vi "test_Update CD XML File.vi"(8 "error in (no error)":errorcluster, 11 "TestCase in":refnum<class "LVLIBP CD XML Updater Unit Tests.lvclass">) -> (0 "error out":errorcluster, 3 "TestCase out":refnum<class "LVLIBP CD XML Updater Unit Tests.lvclass">)   [LabVIEW 2018, in "LVLIBP CD XML Updater Unit Tests.lvclass"]
uses:
  LVLIBP CD XML Updater Unit Tests.lvclass
  <vilib>/addons/_JKI Toolkits/VI Tester/TestCase.llb/TestCase.lvclass
  Utilities/.LVLIBP CD XML Updater/.LVLIBP CD XML Updater.lvlib
  Utilities/.LVLIBP CD XML Updater/Project XML Editor/Project XML Editor.lvclass
  FPGA Addon Test Class/FPGA Addon Test Class.lvclass
  C:/Program Files (x86)/National Instruments/LabVIEW 2018/vi.lib/addons/_JKI Toolkits/VI Tester/TestCase.llb/TestCase.lvclass
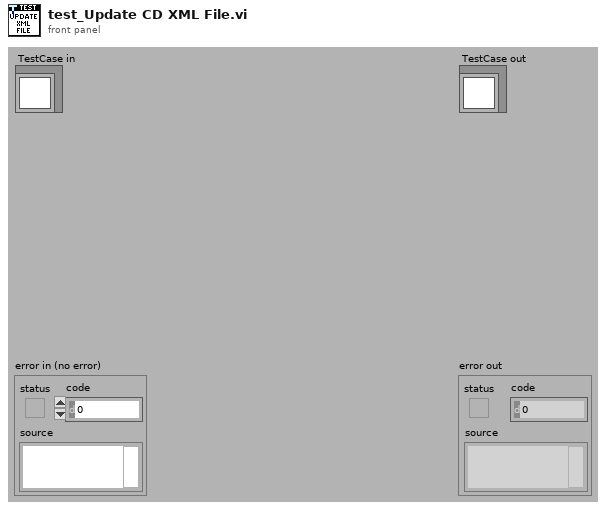
[diagram p1: front panel]
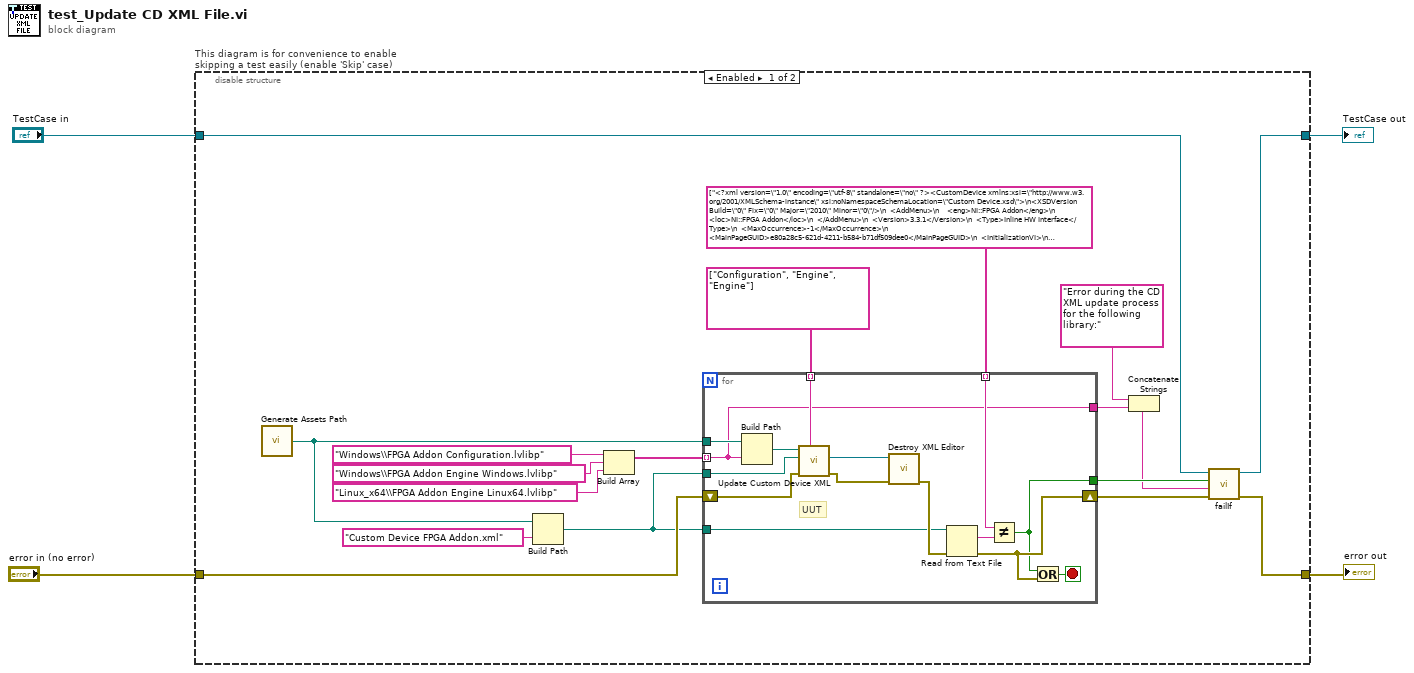
[diagram p0: block diagram]
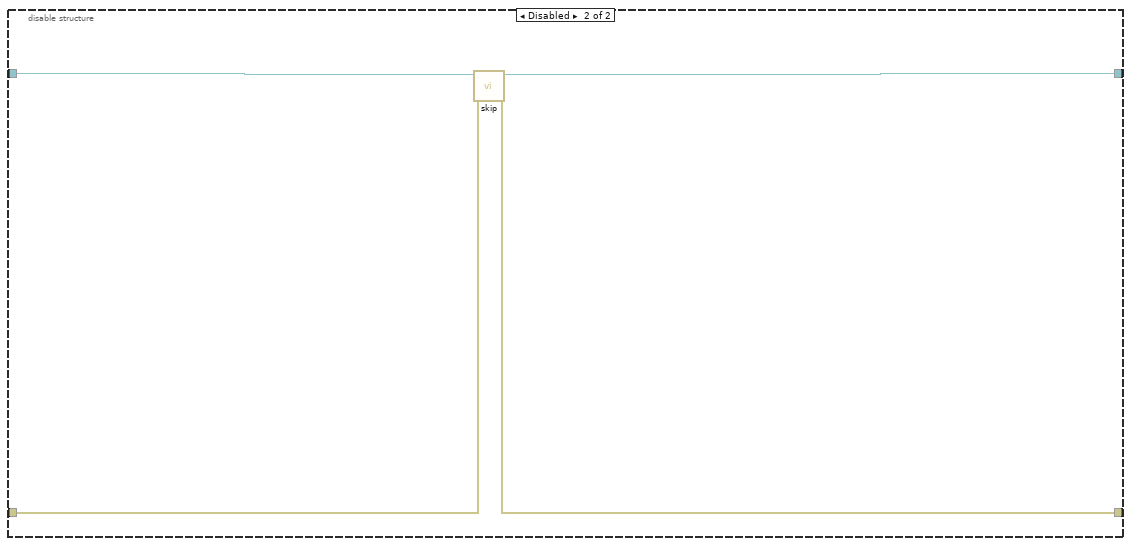
[diagram p2: hidden frame]
diagram:
  n1 = disable-structure "This diagram is for convenience to enable skipping a test easily (enable 'Skip' case)" shown="Enabled" {
    disable-tunnel: "TestCase in" -> [w16 w41]
    disable-tunnel: [w15 w39] -> w1
    disable-tunnel: [w6 w40] -> w3
    disable-tunnel: "error in (no error)" -> [w9 w38]
    frame Enabled {
      n2 = call "Generate Assets Path.vi"() -> ("Assets path"=w11:path)
      n3 = Build Path(base path=w11, name or relative path="Custom Device FPGA Addon.xml") -> (appended path=w5:path)
      n4 = Build Array("Windows\\FPGA Addon Configuration.lvlibp" ("name or relative path"), "Windows\\FPGA Addon Engine Windows.lvlibp" ("name or relative path"), "Linux_x64\\FPGA Addon Engine Linux64.lvlibp" ("name or relative path")) -> (w10:string[])
      n5 = for {
        tunnel: string[] ["Configuration", "Engine", "Engine"] -> [w37] mode=indexing
        tunnel: w5 -> [w36]
        shift-right: [w30] -> w7
        shift-left: w9 -> [w29]
        tunnel: string[] ["<?xml version=\"1.0\" encoding=\"utf-8\" standalone=\"no\" ?><CustomDevice xmlns:xsi=\"http://www.w3.org/2001/XMLSchema-instance\" xsi:noNamespaceSchemaLocation=\"Custom Device.xsd\">\n<XSDVersion Build=\"0\" Fix=\"0\" Major=\"2010\" Minor=\"0\"/>\n  <AddMenu>\n    <eng>NI::FPGA Addon</eng>\n    <loc>NI::FPGA Addon</loc>\n  </AddMenu>\n  <Version>3.3.1</Version>\n  <Type>Inline HW Interface</Type>\n  <MaxOccurrence>-1</MaxOccurrence>\n  <MainPageGUID>e80a28c5-621d-4211-b584-b71df509dee0</MainPageGUID>\n  <InitializationVI>\n    <Type>Action</Type>\n    <Item2Launch>\n      <Type>To Common Doc Dir</Type>\n\t\t<Path>Custom Devices\\FPGA Addon\\Windows\\FPGA Addon Configuration.lvlibp\\Addon\\Addon System Explorer\\Initialization VI.vi</Path>\n    </Item2Launch>\n  </InitializationVI>\n  <CustomDeviceVI>\n\t<SourceDistribution>\n\t\t<Source>\n\t\t\t<SupportedTarget>Windows</SupportedTarget>\n\t\t\t<Source>\n\t\t\t\t<Type>To Common Doc Dir</Type>\n\t\t\t\t<Path>Custom Devices\\FPGA Addon\\Windows\\FPGA Addon Engine Windows.llb\\RT Driver VI.vi</Path>\n\t\t\t</Source>\n\t\t\t<RealTimeSystemDestination>c:\\ni-rt\\VeriStand\\Custom Devices\\FPGA Addon\\FPGA Addon Engine Windows.llb\\RT Driver VI.vi</RealTimeSystemDestination>\n\t\t</Source>\n\t\t<Source>\n\t\t\t<SupportedTarget>Linux_x64</SupportedTarget>\n\t\t\t<Source>\n\t\t\t\t<Type>To Common Doc Dir</Type>\n\t\t\t\t<Path>Custom Devices\\FPGA Addon\\Linux_x64\\FPGA Addon Engine Linux64.llb\\RT Driver VI.vi</Path>\n\t\t\t</Source>\n\t\t\t<RealTimeSystemDestination>c:\\ni-rt\\VeriStand\\Custom Devices\\FPGA Addon\\FPGA Addon Engine Linux64.llb\\RT Driver VI.vi</RealTimeSystemDestination>\n\t\t</Source>\n\t</SourceDistribution>\n\t</CustomDeviceVI>\n  <Dependencies/>\n  <Pages>\n    <Page>\n      <Name>\n        <eng>FPGA Addon</eng>\n        <loc>FPGA Addon</loc>\n      </Name>\n      <GUID>e80a28c5-621d-4211-b584-b71df509dee0</GUID>\n      <Glyph>\n\t\t  \t<Type>To Application Data Dir</Type>\n\t\t\t  <Path>System Explorer\\Glyphs\\fpga device.png</Path>\n\t\t  </Glyph>\n      <Item2Launch>\n        <Type>To Common Doc Dir</Type>\n\t\t    <Path>Custom Devices\\FPGA Addon\\Windows\\FPGA Addon Configuration.lvlibp\\Addon\\Addon System Explorer\\Main Page.vi</Path>\n      </Item2Launch>\n      <RunTimeMenu>\n        <MenuItem>\n          <GUID>01e8f077-156a-4698-bbdc-a047cf741b9d</GUID>\n          <Type>Action</Type>\n          <Name>\n            <eng>Disable</eng>\n            <loc>Disable</loc>\n          </Name>\n          <Item2Launch>\n            <Type>To Common Doc Dir</Type>\n            <Path>Custom Devices\\FPGA Addon\\Windows\\FPGA Addon Configuration.lvlibp\\Addon\\Addon System Explorer\\RTMs\\EnableDisable Main Page.vi</Path>\n          </Item2Launch>\n        </MenuItem>\n        <MenuItem>\n\t\t\t\t\t<GUID>b2ce9074-10ee-4035-b1de-8d57db17ae03</GUID>\n\t\t\t\t\t<Type>Action</Type>\n\t\t\t\t\t<Name>\n\t\t\t\t\t\t<eng>Export Config</eng>\n\t\t\t\t\t\t<loc>Export Config</loc>\n\t\t\t\t\t</Name>\n\t\t\t\t\t<Item2Launch>\n\t\t\t\t\t\t<Type>To Common Doc Dir</Type>\n\t\t\t\t\t\t<Path>Custom Devices\\FPGA Addon\\Windows\\FPGA Addon Configuration.lvlibp\\Addon\\Addon System Explorer\\RTMs\\ExportConfigurationToFile.vi</Path>\n\t\t\t\t\t</Item2Launch>\n\t\t\t\t</MenuItem>\n        <MenuItem>\n          <GUID>7755077A-1485-13A6-5674A23FB86277FF</GUID>\n          <Type>Separator</Type>\n          <Name>\n            <eng>.</eng>\n            <loc>.</loc>\n          </Name>\n          <Item2Launch>\n            <Type>Absolute</Type>\n            <Path>.</Path>\n          </Item2Launch>\n        </MenuItem>\n        <MenuItem>\n          <GUID>77550670-1485-13A6-568B9AB41979630D</GUID>\n          <Type>Action</Type>\n          <Name>\n            <eng>Delete</eng>\n            <loc>Delete</loc>\n          </Name>\n          <Item2Launch>\n            <Type>Absolute</Type>\n            <Path>Actions\\Delete.vi</Path>\n          </Item2Launch>\n        </MenuItem>\n      </RunTimeMenu>\n      <ActionVIOnLoad>\n        <Type>To Common Doc Dir</Type>\n        <Path>Custom Devices\\FPGA Addon\\Windows\\FPGA Addon Configuration.lvlibp\\Addon\\Addon System Explorer\\Actions\\ActionVIOnLoad.vi</Path>\n      </ActionVIOnLoad>\n      <ActionVIOnCompile>\n        <Type>To Common Doc Dir</Type>\n        <Path>Custom Devices\\FPGA Addon\\Windows\\FPGA Addon Configuration.lvlibp\\Addon\\Addon System Explorer\\Actions\\ActionVIOnCompile.vi</Path>\n      </ActionVIOnCompile>\n    </Page>\n    <Page>\n      <Name>\n        <eng>FPGA Addon</eng>\n        <loc>FPGA Addon</loc>\n      </Name>\n      <GUID>1903f8c0-e426-4f25-b8ca-65973b1160fd</GUID>\n      <Glyph>\n        <Type>To Application Data Dir</Type>\n        <Path>System Explorer\\Glyphs\\fpga device_disabled.png</Path>\n      </Glyph>\n      <Item2Launch>\n        <Type>To Common Doc Dir</Type>\n        <Path>Custom Devices\\FPGA Addon\\Windows\\FPGA Addon Configuration.lvlibp\\Addon\\Addon System Explorer\\Main Page.vi</Path>\n      </Item2Launch>\n      <RunTimeMenu>\n        <MenuItem>\n          <GUID>01e8f077-156a-4698-bbdc-a047cf741b9d</GUID>\n          <Type>Action</Type>\n          <Name>\n            <eng>Enable</eng>\n            <loc>Enable</loc>\n          </Name>\n          <Item2Launch>\n            <Type>To Common Doc Dir</Type>\n            <Path>Custom Devices\\FPGA Addon\\Windows\\FPGA Addon Configuration.lvlibp\\Addon\\Addon System Explorer\\RTMs\\EnableDisable Main Page.vi</Path>\n          </Item2Launch>\n        </MenuItem>\n        <MenuItem>\n          <GUID>b2ce9074-10ee-4035-b1de-8d57db17ae03</GUID>\n          <Type>Action</Type>\n          <Name>\n            <eng>Export Config</eng>\n            <loc>Export Config</loc>\n          </Name>\n          <Item2Launch>\n            <Type>To Common Doc Dir</Type>\n            <Path>Custom Devices\\FPGA Addon\\Windows\\FPGA Addon Configuration.lvlibp\\Addon\\Addon System Explorer\\RTMs\\ExportConfigurationToFile.vi</Path>\n          </Item2Launch>\n        </MenuItem>\n        <MenuItem>\n          <GUID>7755077A-1485-13A6-5674A23FB86277FF</GUID>\n          <Type>Separator</Type>\n          <Name>\n            <eng>.</eng>\n            <loc>.</loc>\n          </Name>\n          <Item2Launch>\n            <Type>Absolute</Type>\n            <Path>.</Path>\n          </Item2Launch>\n        </MenuItem>\n        <MenuItem>\n          <GUID>77550670-1485-13A6-568B9AB41979630D</GUID>\n          <Type>Action</Type>\n          <Name>\n            <eng>Delete</eng>\n            <loc>Delete</loc>\n          </Name>\n          <Item2Launch>\n            <Type>Absolute</Type>\n            <Path>Actions\\Delete.vi</Path>\n          </Item2Launch>\n        </MenuItem>\n      </RunTimeMenu>\n      <ActionVIOnLoad>\n        <Type>To Common Doc Dir</Type>\n        <Path>Custom Devices\\FPGA Addon\\Windows\\FPGA Addon Configuration.lvlibp\\Addon\\Addon System Explorer\\Actions\\ActionVIOnLoad.vi</Path>\n      </ActionVIOnLoad>\n    </Page>\n    <Page>\n      <Name>\n        <eng>Scalars</eng>\n        <loc>Scalars</loc>\n      </Name>\n      <DisallowRenaming>true</DisallowRenaming>\n      <DeleteProtection>true</DeleteProtection>\n      <GUID>884b7050-623e-4f2c-925b-6b753ddf9d1a</GUID>\n      <Glyph>\n\t\t  \t<Type>To Application Data Dir</Type>\n\t\t\t  <Path>System Explorer\\Glyphs\\default fpga channel.png</Path>\n\t\t  </Glyph>\n      <Item2Launch>\n        <Type>To Common Doc Dir</Type>\n\t\t    <Path>Custom Devices\\FPGA Addon\\Windows\\FPGA Addon Configuration.lvlibp\\Addon\\Addon System Explorer\\Extra Pages\\Scalars.vi</Path>\n      </Item2Launch>\n      <RunTimeMenu>\n        <MenuItem>\n          <GUID>03D3BE0A-1485-13A6-563AEB9BF271825A</GUID>\n          <Type>VI</Type>\n          <MinNrOfChilds>1</MinNrOfChilds>\n          <Name>\n            <eng>Delete Multiple Items</eng>\n            <loc>Delete Multiple Items</loc>\n          </Name>\n          <Item2Launch>\n            <Type>Absolute</Type>\n            <Path>Dialogs\\Delete Multiple Items.vi</Path>\n          </Item2Launch>\n        </MenuItem>    \n      </RunTimeMenu>\n    </Page>\n    <Page>\n      <Name>\n        <eng>Scalar Inputs</eng>\n        <loc>Scalar Inputs</loc>\n      </Name>\n      <DisallowRenaming>true</DisallowRenaming>\n      <DeleteProtection>true</DeleteProtection>\n      <GUID>45f50bc5-dab3-4e15-b99b-0f8c8c0fe0f0</GUID>\n      <Glyph>\n\t\t  \t<Type>To Application Data Dir</Type>\n\t\t  \t<Path>System Explorer\\Glyphs\\ChnGroup.png</Path>\n\t\t  </Glyph>\n      <Item2Launch>\n        <Type>To Common Doc Dir</Type>\n\t\t    <Path>Custom Devices\\FPGA Addon\\Windows\\FPGA Addon Configuration.lvlibp\\Addon\\Addon System Explorer\\Extra Pages\\Scalar Inputs.vi</Path>\n      </Item2Launch>\n    </Page>\n    <Page>\n      <Name>\n        <eng>Group Input</eng>\n        <loc>Group Input</loc>\n      </Name>\n      <GUID>88748f7d-ce11-4328-8f35-56fd574a40c1</GUID>\n      <Glyph>\n        <Type>To Common Doc Dir</Type>\n\t\t    <Path>Custom Devices\\FPGA Addon\\Windows\\Glyphs\\Group.png</Path>\n\t\t  </Glyph>\n      <Item2Launch>\n        <Type>To Common Doc Dir</Type>\n\t\t    <Path>Custom Devices\\FPGA Addon\\Windows\\FPGA Addon Configuration.lvlibp\\Addon\\Addon System Explorer\\Extra Pages\\Scalar Inputs.vi</Path>\n      </Item2Launch>\n    </Page>\n    <Page>\n      <Name>\n        <eng>Scalar Outputs</eng>\n        <loc>Scalar Outputs</loc>\n      </Name>\n      <DisallowRenaming>true</DisallowRenaming>\n      <DeleteProtection>true</DeleteProtection>\n      <GUID>7d46fed9-731a-4423-8f13-aa8ac2cd791c</GUID>\n      <Glyph>\n\t\t\t  <Type>To Application Data Dir</Type>\n\t\t\t  <Path>System Explorer\\Glyphs\\ChnGroup.png</Path>\n\t\t  </Glyph>\n      <Item2Launch>\n        <Type>To Common Doc Dir</Type>\n\t\t    <Path>Custom Devices\\FPGA Addon\\Windows\\FPGA Addon Configuration.lvlibp\\Addon\\Addon System Explorer\\Extra Pages\\Scalar Outputs.vi</Path>\n      </Item2Launch>\n    </Page>\n    <Page>\n      <Name>\n        <eng>Group Output</eng>\n        <loc>Group Output</loc>\n      </Name>\n      <GUID>58901a15-a42e-477a-af06-3ceeb84f52de</GUID>\n      <Glyph>\n        <Type>To Common Doc Dir</Type>\n\t\t    <Path>Custom Devices\\FPGA Addon\\Windows\\Glyphs\\Group.png</Path>\n\t\t  </Glyph>\n      <Item2Launch>\n        <Type>To Common Doc Dir</Type>\n\t\t    <Path>Custom Devices\\FPGA Addon\\Windows\\FPGA Addon Configuration.lvlibp\\Addon\\Addon System Explorer\\Extra Pages\\Scalar Outputs.vi</Path>\n      </Item2Launch>\n    </Page>\n    <Page>\n      <Name>\n        <eng>Waveforms</eng>\n        <loc>Waveforms</loc>\n      </Name>\n      <DisallowRenaming>true</DisallowRenaming>\n      <DeleteProtection>true</DeleteProtection>\n      <GUID>5f75895a-bfdb-4cd8-9ef2-787e261eba38</GUID>\n      <Glyph>\n\t\t\t  <Type>To Application Data Dir</Type>\n\t\t\t  <Path>System Explorer\\Glyphs\\waveform.png</Path>\n\t\t  </Glyph>\n      <Item2Launch>\n        <Type>To Common Doc Dir</Type>\n\t\t    <Path>Custom Devices\\FPGA Addon\\Windows\\FPGA Addon Configuration.lvlibp\\Addon\\Addon System Explorer\\Extra Pages\\Waveforms.vi</Path>\n      </Item2Launch>\n      <RunTimeMenu>\n        <MenuItem>\n          <GUID>03D3BE0A-1485-13A6-563AEB9BF271825A</GUID>\n          <Type>VI</Type>\n          <MinNrOfChilds>1</MinNrOfChilds>\n          <Name>\n            <eng>Delete Multiple Items</eng>\n            <loc>Delete Multiple Items</loc>\n          </Name>\n          <Item2Launch>\n            <Type>Absolute</Type>\n            <Path>Dialogs\\Delete Multiple Items.vi</Path>\n          </Item2Launch>\n        </MenuItem>\n      </RunTimeMenu>\n    </Page>\n    <Page>\n      <Name>\n        <eng>Waveform Inputs</eng>\n        <loc>Waveform Inputs</loc>\n      </Name>\n      <DisallowRenaming>true</DisallowRenaming>\n      <DeleteProtection>true</DeleteProtection>\n      <ExcludeFromAlphabeticalOrder>true</ExcludeFromAlphabeticalOrder>\n      <GUID>165959cb-b691-43bd-9f8b-54fe62f4b534</GUID>\n      <Glyph>\n\t\t\t  <Type>To Application Data Dir</Type>\n\t\t\t  <Path>System Explorer\\Glyphs\\ChnGroup.png</Path>\n\t\t  </Glyph>\n      <Item2Launch>\n        <Type>To Common Doc Dir</Type>\n\t\t    <Path>Custom Devices\\FPGA Addon\\Windows\\FPGA Addon Configuration.lvlibp\\Addon\\Addon System Explorer\\Extra Pages\\Waveform Inputs.vi</Path>\n      </Item2Launch>\n    </Page>\n    <Page>\n      <Name>\n        <eng>Waveform Outputs</eng>\n        <loc>Waveform Outputs</loc>\n      </Name>\n      <DisallowRenaming>true</DisallowRenaming>\n      <DeleteProtection>true</DeleteProtection>\n      <ExcludeFromAlphabeticalOrder>true</ExcludeFromAlphabeticalOrder>\n      <GUID>bc66db3e-ace6-4d58-add4-89e89e885df7</GUID>\n      <Glyph>\n        <Type>To Application Data Dir</Type>\n        <Path>System Explorer\\Glyphs\\ChnGroup.png</Path>\n      </Glyph>\n      <Item2Launch>\n        <Type>To Common Doc Dir</Type>\n        <Path>Custom Devices\\FPGA Addon\\Windows\\FPGA Addon Configuration.lvlibp\\Addon\\Addon System Explorer\\Extra Pages\\Waveform Outputs.vi</Path>\n      </Item2Launch>\n    </Page>\n    <Page>\n      <Name>\n        <eng>Scalar Input</eng>\n        <loc>Scalar Input</loc>\n      </Name>\n      <GUID>9bd0c044-925c-4d1d-a44e-de3c4043858c</GUID>\n      <Glyph>\n\t\t  \t<Type>To Application Data Dir</Type>\n\t\t  \t<Path>System Explorer\\Glyphs\\default fpga channel.png</Path>\n\t\t  </Glyph>\n      <Item2Launch>\n        <Type>To Common Doc Dir</Type>\n\t\t    <Path>Custom Devices\\FPGA Addon\\Windows\\FPGA Addon Configuration.lvlibp\\Addon\\Addon System Explorer\\Extra Pages\\Scalar Input.vi</Path>\n      </Item2Launch>\n      <RunTimeMenu>\n        <MenuItem>\n          <GUID>2cd33a82-ccc0-4cb3-affc-1385b5dc0dd8</GUID>\n          <Type>Action</Type>\n          <Name>\n            <eng>Enable Bitpacked</eng>\n            <loc>Enable Bitpacked</loc>\n          </Name>\n          <Item2Launch>\n            <Type>To Common Doc Dir</Type>\n            <Path>Custom Devices\\FPGA Addon\\Windows\\FPGA Addon Configuration.lvlibp\\Addon\\Addon System Explorer\\RTMs\\Switch Scalar Type.vi</Path>\n          </Item2Launch>\n        </MenuItem>\n        <MenuItem>\n          <GUID>7755077A-1485-13A6-5674A23FB86277FF</GUID>\n          <Type>Separator</Type>\n          <Name>\n            <eng>.</eng>\n            <loc>.</loc>\n          </Name>\n          <Item2Launch>\n            <Type>Absolute</Type>\n            <Path>.</Path>\n          </Item2Launch>\n        </MenuItem>\n        <MenuItem>\n          <GUID>77550670-1485-13A6-568B9AB41979630D</GUID>\n          <Type>Action</Type>\n          <Name>\n            <eng>Delete</eng>\n            <loc>Delete</loc>\n          </Name>\n          <Item2Launch>\n            <Type>Absolute</Type>\n            <Path>Actions\\Delete.vi</Path>\n          </Item2Launch>\n        </MenuItem>\n      </RunTimeMenu>\n    </Page>\n    <Page>\n      <Name>\n        <eng>Scalar Output</eng>\n        <loc>Scalar Output</loc>\n      </Name>\n      <GUID>625afbbf-e929-46eb-93d1-fe7033ba1e7b</GUID>\n      <Glyph>\n\t\t  \t<Type>To Application Data Dir</Type>\n\t\t  \t<Path>System Explorer\\Glyphs\\default fpga channel.png</Path>\n\t  \t</Glyph>\n      <Item2Launch>\n        <Type>To Common Doc Dir</Type>\n\t\t    <Path>Custom Devices\\FPGA Addon\\Windows\\FPGA Addon Configuration.lvlibp\\Addon\\Addon System Explorer\\Extra Pages\\Scalar Output.vi</Path>\n      </Item2Launch>\n      <RunTimeMenu>\n        <MenuItem>\n          <GUID>2cd33a82-ccc0-4cb3-affc-1385b5dc0dd8</GUID>\n          <Type>Action</Type>\n          <Name>\n            <eng>Enable Bitpacked</eng>\n            <loc>Enable Bitpacked</loc>\n          </Name>\n          <Item2Launch>\n            <Type>To Common Doc Dir</Type>\n            <Path>Custom Devices\\FPGA Addon\\Windows\\FPGA Addon Configuration.lvlibp\\Addon\\Addon System Explorer\\RTMs\\Switch Scalar Type.vi</Path>\n          </Item2Launch>\n        </MenuItem>\n        <MenuItem>\n          <GUID>7755077A-1485-13A6-5674A23FB86277FF</GUID>\n          <Type>Separator</Type>\n          <Name>\n            <eng>.</eng>\n            <loc>.</loc>\n          </Name>\n          <Item2Launch>\n            <Type>Absolute</Type>\n            <Path>.</Path>\n          </Item2Launch>\n        </MenuItem>\n        <MenuItem>\n          <GUID>77550670-1485-13A6-568B9AB41979630D</GUID>\n          <Type>Action</Type>\n          <Name>\n            <eng>Delete</eng>\n            <loc>Delete</loc>\n          </Name>\n          <Item2Launch>\n            <Type>Absolute</Type>\n            <Path>Actions\\Delete.vi</Path>\n          </Item2Launch>\n        </MenuItem>\n      </RunTimeMenu>\n    </Page>\n    <Page>\n      <Name>\n        <eng>DMA</eng>\n        <loc>DMA</loc>\n      </Name>\n      <ExcludeFromAlphabeticalOrder>true</ExcludeFromAlphabeticalOrder>\n      <GUID>fdfaa619-d09f-452b-8143-c1a261c13b7a</GUID>\n      <Glyph>\n\t\t\t  <Type>To Application Data Dir</Type>\n\t\t\t  <Path>System Explorer\\Glyphs\\Lookup Table.png</Path>\n\t\t  </Glyph>\n      <Item2Launch>\n        <Type>To Common Doc Dir</Type>\n\t\t    <Path>Custom Devices\\FPGA Addon\\Windows\\FPGA Addon Configuration.lvlibp\\Addon\\Addon System Explorer\\Extra Pages\\DMA Channel.vi</Path>\n      </Item2Launch>\n      <RunTimeMenu>\n         <MenuItem>\n            <GUID>345ad323-e622-4d27-9f97-b3d588c29827</GUID>\n            <Type>Action</Type>\n            <Name>\n              <eng>Import DMA Channels</eng>\n              <loc>Import DMA Channels</loc>\n            </Name>\n            <Item2Launch>\n              <Type>To Common Doc Dir</Type>\n              <Path>Custom Devices\\FPGA Addon\\Windows\\FPGA Addon Configuration.lvlibp\\Addon\\Addon System Explorer\\RTMs\\Import DMA Channels RTM.vi</Path>\n            </Item2Launch>\n          </MenuItem>\n          <MenuItem>\n            <GUID>7755077A-1485-13A6-5674A23FB86277FF</GUID>\n            <Type>Separator</Type>\n            <Name>\n              <eng>.</eng>\n              <loc>.</loc>\n            </Name>\n            <Item2Launch>\n              <Type>Absolute</Type>\n              <Path>.</Path>\n            </Item2Launch>\n          </MenuItem>\n      </RunTimeMenu>\n    <ButtonList>\n        <Button>\n          <ID>Import DMA Channels</ID>\n          <Glyph>\n            <Type>To Application Data Dir</Type>\n            <Path>System Explorer\\Glyphs\\NI-XNET ImportXNETFrames.png</Path>\n          </Glyph>\n          <Type>Action</Type>\n          <ReferencedGUID>345ad323-e622-4d27-9f97-b3d588c29827</ReferencedGUID>\n          <ButtonText>\n            <eng>Import DMA Channels</eng>\n            <loc>Import DMA Channels</loc>\n          </ButtonText>\n          <Caption>\n            <eng>Import DMA Channels</eng>\n            <loc>Import DMA Channels</loc>\n          </Caption>\n          <TipStrip>\n            <eng>Import DMA Channels</eng>\n            <loc>Import DMA Channels</loc>\n          </TipStrip>\n          <Documentation>\n            <eng/>\n            <loc/>\n          </Documentation>\n        </Button>\n    </ButtonList>\n    </Page>\n    <Page>\n      <Name>\n        <eng>Waveform Output</eng>\n        <loc>Waveform Output</loc>\n      </Name>\n      <DeleteProtection>true</DeleteProtection>\n      <ExcludeFromAlphabeticalOrder>true</ExcludeFromAlphabeticalOrder>\n      <GUID>0c0ecc88-7768-47db-a589-856e32a93156</GUID>\n      <Glyph>\n        <Type>To Application Data Dir</Type>\n        <Path>System Explorer\\Glyphs\\waveform.png</Path>\n      </Glyph>\n      <Item2Launch>\n        <Type>To Common Doc Dir</Type>\n        <Path>Custom Devices\\FPGA Addon\\Windows\\FPGA Addon Configuration.lvlibp\\Addon\\Addon System Explorer\\Extra Pages\\Waveform Output.vi</Path>\n      </Item2Launch>\n    </Page>\n    <Page>\n      <Name>\n        <eng>Waveform Input</eng>\n        <loc>Waveform Input</loc>\n      </Name>\n      <DeleteProtection>true</DeleteProtection>\n      <ExcludeFromAlphabeticalOrder>true</ExcludeFromAlphabeticalOrder>\n      <GUID>2afc1de4-b056-47bb-a2ad-eec5ad0d30b6</GUID>\n      <Glyph>\n        <Type>To Application Data Dir</Type>\n        <Path>System Explorer\\Glyphs\\waveform.png</Path>\n      </Glyph>\n      <Item2Launch>\n        <Type>To Common Doc Dir</Type>\n        <Path>Custom Devices\\FPGA Addon\\Windows\\FPGA Addon Configuration.lvlibp\\Addon\\Addon System Explorer\\Extra Pages\\Waveform Input.vi</Path>\n      </Item2Launch>\n    </Page>\n    <Page>\n      <Name>\n        <eng>DMA Status Channels</eng>\n        <loc>DMA Status Channels</loc>\n      </Name>\n      <DisallowRenaming>true</DisallowRenaming>\n      <DeleteProtection>true</DeleteProtection>\n      <ExcludeFromAlphabeticalOrder>true</ExcludeFromAlphabeticalOrder>\n      <GUID>4e1a084b-2b8b-4128-8417-f0007d9ffe93</GUID>\n      <Glyph>\n\t\t  \t<Type>To Application Data Dir</Type>\n\t\t  \t<Path>System Explorer\\Glyphs\\event-based.png</Path>\n\t\t  </Glyph>\n      <Item2Launch>\n        <Type>To Common Doc Dir</Type>\n\t    \t<Path>Custom Devices\\FPGA Addon\\Windows\\FPGA Addon Configuration.lvlibp\\Addon\\Addon System Explorer\\Extra Pages\\DMA Status Channels.vi</Path>\n      </Item2Launch>\n    </Page>\n    <Page>\n      <Name>\n        <eng>DMA Error</eng>\n        <loc>DMA Error</loc>\n      </Name>\n      <DisallowRenaming>true</DisallowRenaming>\n      <DeleteProtection>true</DeleteProtection>\n      <GUID>708ff167-b4eb-405e-bb0f-5c2fb305da21</GUID>\n      <Glyph>\n        <Type>To Application Data Dir</Type>\n        <Path>System Explorer\\Glyphs\\RM Information Channels.png</Path>\n      </Glyph>\n      <Item2Launch>\n        <Type>To Common Doc Dir</Type>\n        <Path>Custom Devices\\FPGA Addon\\Windows\\FPGA Addon Configuration.lvlibp\\Addon\\Addon System Explorer\\Extra Pages\\DMA Error.vi</Path>\n      </Item2Launch>\n    </Page>\n    <Page>\n      <Name>\n        <eng>DMA Elements Remaining</eng>\n        <loc>DMA Elements Remaining</loc>\n      </Name>\n      <DisallowRenaming>true</DisallowRenaming>\n      <DeleteProtection>true</DeleteProtection>\n      <GUID>785497d1-fc1e-46c9-8feb-aa61f2850cff</GUID>\n      <Glyph>\n        <Type>To Application Data Dir</Type>\n        <Path>System Explorer\\Glyphs\\RM Information Channels.png</Path>\n      </Glyph>\n      <Item2Launch>\n        <Type>To Common Doc Dir</Type>\n        <Path>Custom Devices\\FPGA Addon\\Windows\\FPGA Addon Configuration.lvlibp\\Addon\\Addon System Explorer\\Extra Pages\\DMA Elements Remaining.vi</Path>\n      </Item2Launch>\n    </Page>\n    <Page>\n      <Name>\n        <eng>Scalar Input Bitpacked</eng>\n        <loc>Scalar Input Bitpacked</loc>\n      </Name>\n      <ExcludeFromAlphabeticalOrder>true</ExcludeFromAlphabeticalOrder>\n      <GUID>8489bf21-57e3-4e68-bdd5-eadff573ec1e</GUID>\n      <Glyph>\n        <Type>To Common Doc Dir</Type>\n\t\t  <Path>Custom Devices\\FPGA Addon\\Windows\\Glyphs\\Bitpacked.png</Path>\n      </Glyph>\n      <Item2Launch>\n        <Type>To Common Doc Dir</Type>\n        <Path>Custom Devices\\FPGA Addon\\Windows\\FPGA Addon Configuration.lvlibp\\Addon\\Addon System Explorer\\Extra Pages\\Scalar Bitpacked.vi</Path>\n      </Item2Launch>\n      <RunTimeMenu>\n        <MenuItem>\n          <GUID>2cd33a82-ccc0-4cb3-affc-1385b5dc0dd8</GUID>\n          <Type>Action</Type>\n          <Name>\n            <eng>Disable Bitpacked</eng>\n            <loc>Disable Bitpacked</loc>\n          </Name>\n          <Item2Launch>\n            <Type>To Common Doc Dir</Type>\n            <Path>Custom Devices\\FPGA Addon\\Windows\\FPGA Addon Configuration.lvlibp\\Addon\\Addon System Explorer\\RTMs\\Switch Scalar Type.vi</Path>\n          </Item2Launch>\n        </MenuItem>\n        <MenuItem>\n          <GUID>7755077A-1485-13A6-5674A23FB86277FF</GUID>\n          <Type>Separator</Type>\n          <Name>\n            <eng>.</eng>\n            <loc>.</loc>\n          </Name>\n          <Item2Launch>\n            <Type>Absolute</Type>\n            <Path>.</Path>\n          </Item2Launch>\n        </MenuItem>\n        <MenuItem>\n          <GUID>77550670-1485-13A6-568B9AB41979630D</GUID>\n          <Type>Action</Type>\n          <Name>\n            <eng>Delete</eng>\n            <loc>Delete</loc>\n          </Name>\n          <Item2Launch>\n            <Type>Absolute</Type>\n            <Path>Actions\\Delete.vi</Path>\n          </Item2Launch>\n        </MenuItem>\n      </RunTimeMenu>\n    </Page>\n    <Page>\n      <Name>\n        <eng>Scalar Output Bitpacked</eng>\n        <loc>Scalar Output Bitpacked</loc>\n      </Name>\n      <ExcludeFromAlphabeticalOrder>true</ExcludeFromAlphabeticalOrder>\n      <GUID>ebfc3e29-7579-49df-b828-0da2c3787b5f</GUID>\n      <Glyph>\n        <Type>To Common Doc Dir</Type>\n\t\t  <Path>Custom Devices\\FPGA Addon\\Windows\\Glyphs\\Bitpacked.png</Path>\n      </Glyph>\n      <Item2Launch>\n        <Type>To Common Doc Dir</Type>\n        <Path>Custom Devices\\FPGA Addon\\Windows\\FPGA Addon Configuration.lvlibp\\Addon\\Addon System Explorer\\Extra Pages\\Scalar Bitpacked.vi</Path>\n      </Item2Launch>\n      <RunTimeMenu>\n        <MenuItem>\n          <GUID>2cd33a82-ccc0-4cb3-affc-1385b5dc0dd8</GUID>\n          <Type>Action</Type>\n          <Name>\n            <eng>Disable Bitpacked</eng>\n            <loc>Disable Bitpacked</loc>\n          </Name>\n          <Item2Launch>\n            <Type>To Common Doc Dir</Type>\n            <Path>Custom Devices\\FPGA Addon\\Windows\\FPGA Addon Configuration.lvlibp\\Addon\\Addon System Explorer\\RTMs\\Switch Scalar Type.vi</Path>\n          </Item2Launch>\n        </MenuItem>\n        <MenuItem>\n          <GUID>7755077A-1485-13A6-5674A23FB86277FF</GUID>\n          <Type>Separator</Type>\n          <Name>\n            <eng>.</eng>\n            <loc>.</loc>\n          </Name>\n          <Item2Launch>\n            <Type>Absolute</Type>\n            <Path>.</Path>\n          </Item2Launch>\n        </MenuItem>\n        <MenuItem>\n          <GUID>77550670-1485-13A6-568B9AB41979630D</GUID>\n          <Type>Action</Type>\n          <Name>\n            <eng>Delete</eng>\n            <loc>Delete</loc>\n          </Name>\n          <Item2Launch>\n            <Type>Absolute</Type>\n            <Path>Actions\\Delete.vi</Path>\n          </Item2Launch>\n        </MenuItem>\n      </RunTimeMenu>\n    </Page>\n    <Page>\n      <Name>\n        <eng>Bitpacked Input</eng>\n        <loc>Bitpacked Input</loc>\n      </Name>\n      <DeleteProtection>true</DeleteProtection>\n      <ExcludeFromAlphabeticalOrder>true</ExcludeFromAlphabeticalOrder>\n      <GUID>4b03cffd-e469-431a-ba96-aca85ece66af</GUID>\n      <Glyph>\n        <Type>To Application Data Dir</Type>\n        <Path>System Explorer\\Glyphs\\default fpga channel.png</Path>\n      </Glyph>\n      <Item2Launch>\n        <Type>To Common Doc Dir</Type>\n        <Path>Custom Devices\\FPGA Addon\\Windows\\FPGA Addon Configuration.lvlibp\\Addon\\Addon System Explorer\\Extra Pages\\Scalar Input.vi</Path>\n      </Item2Launch>\n    </Page>\n    <Page>\n      <Name>\n        <eng>Bitpacked Output</eng>\n        <loc>Bitpacked Output</loc>\n      </Name>\n      <DeleteProtection>true</DeleteProtection>\n      <ExcludeFromAlphabeticalOrder>true</ExcludeFromAlphabeticalOrder>\n      <GUID>6db3f02b-654f-4ed6-bd84-80bb5242a557</GUID>\n      <Glyph>\n        <Type>To Application Data Dir</Type>\n        <Path>System Explorer\\Glyphs\\default fpga channel.png</Path>\n      </Glyph>\n      <Item2Launch>\n        <Type>To Common Doc Dir</Type>\n        <Path>Custom Devices\\FPGA Addon\\Windows\\FPGA Addon Configuration.lvlibp\\Addon\\Addon System Explorer\\Extra Pages\\Scalar Output.vi</Path>\n      </Item2Launch>\n    </Page>\n      <Page>\n      <Name>\n        <eng>Static Scalar Input</eng>\n        <loc>Static Scalar Input</loc>\n      </Name>\n      <GUID>7579cb69-d559-4b2b-a1fc-0d112e8661b6</GUID>\n      <Glyph>\n        <Type>To Application Data Dir</Type>\n        <Path>System Explorer\\Glyphs\\default fpga channel.png</Path>\n      </Glyph>\n      <Item2Launch>\n        <Type>To Common Doc Dir</Type>\n        <Path>Custom Devices\\FPGA Addon\\Windows\\FPGA Addon Configuration.lvlibp\\Addon\\Addon System Explorer\\Extra Pages\\Scalar Input.vi</Path>\n      </Item2Launch>\n      <RunTimeMenu>\n        <MenuItem>\n          <GUID>77550670-1485-13A6-568B9AB41979630D</GUID>\n          <Type>Action</Type>\n          <Name>\n            <eng>Delete</eng>\n            <loc>Delete</loc>\n          </Name>\n          <Item2Launch>\n            <Type>Absolute</Type>\n            <Path>Actions\\Delete.vi</Path>\n          </Item2Launch>\n        </MenuItem>\n      </RunTimeMenu>\n    </Page>\n    <Page>\n      <Name>\n        <eng>Static Scalar Output</eng>\n        <loc>Static Scalar Output</loc>\n      </Name>\n      <GUID>ddc5186b-4b14-4629-b48a-cef4575f789c</GUID>\n      <Glyph>\n        <Type>To Application Data Dir</Type>\n        <Path>System Explorer\\Glyphs\\default fpga channel.png</Path>\n      </Glyph>\n      <Item2Launch>\n        <Type>To Common Doc Dir</Type>\n        <Path>Custom Devices\\FPGA Addon\\Windows\\FPGA Addon Configuration.lvlibp\\Addon\\Addon System Explorer\\Extra Pages\\Scalar Output.vi</Path>\n      </Item2Launch>\n      <RunTimeMenu>\n        <MenuItem>\n          <GUID>77550670-1485-13A6-568B9AB41979630D</GUID>\n          <Type>Action</Type>\n          <Name>\n            <eng>Delete</eng>\n            <loc>Delete</loc>\n          </Name>\n          <Item2Launch>\n            <Type>Absolute</Type>\n            <Path>Actions\\Delete.vi</Path>\n          </Item2Launch>\n        </MenuItem>\n      </RunTimeMenu>\n    </Page>\n      <Page>\n      <Name>\n        <eng>Speciality IO</eng>\n        <loc>Speciality IO</loc>\n      </Name>\n      <ExcludeFromAlphabeticalOrder>true</ExcludeFromAlphabeticalOrder>\n      <GUID>25832021-24b6-475a-aa84-f4ed7870ed99</GUID>\n      <Glyph>\n        <Type>To Common Doc Dir</Type>\n\t\t  <Path>Custom Devices\\FPGA Addon\\Windows\\Glyphs\\IP Core.png</Path>\n      </Glyph>\n      <Item2Launch>\n        <Type>To Common Doc Dir</Type>\n        <Path>Custom Devices\\FPGA Addon\\Windows\\FPGA Addon Configuration.lvlibp\\Addon\\Addon System Explorer\\Extra Pages\\Speciality IO.vi</Path>\n      </Item2Launch>\n    </Page>\n  </Pages>\n  <CustomXML>\n    <Dummy/>\n  </CustomXML>\n</CustomDevice>", "<?xml version=\"1.0\" encoding=\"utf-8\" standalone=\"no\" ?><CustomDevice xmlns:xsi=\"http://www.w3.org/2001/XMLSchema-instance\" xsi:noNamespaceSchemaLocation=\"Custom Device.xsd\">\n<XSDVersion Build=\"0\" Fix=\"0\" Major=\"2010\" Minor=\"0\"/>\n  <AddMenu>\n    <eng>NI::FPGA Addon</eng>\n    <loc>NI::FPGA Addon</loc>\n  </AddMenu>\n  <Version>3.3.1</Version>\n  <Type>Inline HW Interface</Type>\n  <MaxOccurrence>-1</MaxOccurrence>\n  <MainPageGUID>e80a28c5-621d-4211-b584-b71df509dee0</MainPageGUID>\n  <InitializationVI>\n    <Type>Action</Type>\n    <Item2Launch>\n      <Type>To Common Doc Dir</Type>\n\t\t<Path>Custom Devices\\FPGA Addon\\Windows\\FPGA Addon Configuration.lvlibp\\Addon\\Addon System Explorer\\Initialization VI.vi</Path>\n    </Item2Launch>\n  </InitializationVI>\n  <CustomDeviceVI>\n\t<SourceDistribution>\n\t\t<Source>\n\t\t\t<SupportedTarget>Windows</SupportedTarget>\n\t\t\t<Source>\n\t\t\t\t<Type>To Common Doc Dir</Type>\n\t\t\t\t<Path>Custom Devices\\FPGA Addon\\Windows\\FPGA Addon Engine Windows.lvlibp\\Addon\\Addon Engine\\RT Driver VI.vi</Path>\n\t\t\t</Source>\n\t\t\t<RealTimeSystemDestination>c:\\ni-rt\\VeriStand\\Custom Devices\\FPGA Addon\\FPGA Addon Engine Windows.lvlibp\\Addon\\Addon Engine\\RT Driver VI.vi</RealTimeSystemDestination>\n\t\t</Source>\n\t\t<Source>\n\t\t\t<SupportedTarget>Linux_x64</SupportedTarget>\n\t\t\t<Source>\n\t\t\t\t<Type>To Common Doc Dir</Type>\n\t\t\t\t<Path>Custom Devices\\FPGA Addon\\Linux_x64\\FPGA Addon Engine Linux64.llb\\RT Driver VI.vi</Path>\n\t\t\t</Source>\n\t\t\t<RealTimeSystemDestination>c:\\ni-rt\\VeriStand\\Custom Devices\\FPGA Addon\\FPGA Addon Engine Linux64.llb\\RT Driver VI.vi</RealTimeSystemDestination>\n\t\t</Source>\n\t</SourceDistribution>\n\t</CustomDeviceVI>\n  <Dependencies/>\n  <Pages>\n    <Page>\n      <Name>\n        <eng>FPGA Addon</eng>\n        <loc>FPGA Addon</loc>\n      </Name>\n      <GUID>e80a28c5-621d-4211-b584-b71df509dee0</GUID>\n      <Glyph>\n\t\t  \t<Type>To Application Data Dir</Type>\n\t\t\t  <Path>System Explorer\\Glyphs\\fpga device.png</Path>\n\t\t  </Glyph>\n      <Item2Launch>\n        <Type>To Common Doc Dir</Type>\n\t\t    <Path>Custom Devices\\FPGA Addon\\Windows\\FPGA Addon Configuration.lvlibp\\Addon\\Addon System Explorer\\Main Page.vi</Path>\n      </Item2Launch>\n      <RunTimeMenu>\n        <MenuItem>\n          <GUID>01e8f077-156a-4698-bbdc-a047cf741b9d</GUID>\n          <Type>Action</Type>\n          <Name>\n            <eng>Disable</eng>\n            <loc>Disable</loc>\n          </Name>\n          <Item2Launch>\n            <Type>To Common Doc Dir</Type>\n            <Path>Custom Devices\\FPGA Addon\\Windows\\FPGA Addon Configuration.lvlibp\\Addon\\Addon System Explorer\\RTMs\\EnableDisable Main Page.vi</Path>\n          </Item2Launch>\n        </MenuItem>\n        <MenuItem>\n\t\t\t\t\t<GUID>b2ce9074-10ee-4035-b1de-8d57db17ae03</GUID>\n\t\t\t\t\t<Type>Action</Type>\n\t\t\t\t\t<Name>\n\t\t\t\t\t\t<eng>Export Config</eng>\n\t\t\t\t\t\t<loc>Export Config</loc>\n\t\t\t\t\t</Name>\n\t\t\t\t\t<Item2Launch>\n\t\t\t\t\t\t<Type>To Common Doc Dir</Type>\n\t\t\t\t\t\t<Path>Custom Devices\\FPGA Addon\\Windows\\FPGA Addon Configuration.lvlibp\\Addon\\Addon System Explorer\\RTMs\\ExportConfigurationToFile.vi</Path>\n\t\t\t\t\t</Item2Launch>\n\t\t\t\t</MenuItem>\n        <MenuItem>\n          <GUID>7755077A-1485-13A6-5674A23FB86277FF</GUID>\n          <Type>Separator</Type>\n          <Name>\n            <eng>.</eng>\n            <loc>.</loc>\n          </Name>\n          <Item2Launch>\n            <Type>Absolute</Type>\n            <Path>.</Path>\n          </Item2Launch>\n        </MenuItem>\n        <MenuItem>\n          <GUID>77550670-1485-13A6-568B9AB41979630D</GUID>\n          <Type>Action</Type>\n          <Name>\n            <eng>Delete</eng>\n            <loc>Delete</loc>\n          </Name>\n          <Item2Launch>\n            <Type>Absolute</Type>\n            <Path>Actions\\Delete.vi</Path>\n          </Item2Launch>\n        </MenuItem>\n      </RunTimeMenu>\n      <ActionVIOnLoad>\n        <Type>To Common Doc Dir</Type>\n        <Path>Custom Devices\\FPGA Addon\\Windows\\FPGA Addon Configuration.lvlibp\\Addon\\Addon System Explorer\\Actions\\ActionVIOnLoad.vi</Path>\n      </ActionVIOnLoad>\n      <ActionVIOnCompile>\n        <Type>To Common Doc Dir</Type>\n        <Path>Custom Devices\\FPGA Addon\\Windows\\FPGA Addon Configuration.lvlibp\\Addon\\Addon System Explorer\\Actions\\ActionVIOnCompile.vi</Path>\n      </ActionVIOnCompile>\n    </Page>\n    <Page>\n      <Name>\n        <eng>FPGA Addon</eng>\n        <loc>FPGA Addon</loc>\n      </Name>\n      <GUID>1903f8c0-e426-4f25-b8ca-65973b1160fd</GUID>\n      <Glyph>\n        <Type>To Application Data Dir</Type>\n        <Path>System Explorer\\Glyphs\\fpga device_disabled.png</Path>\n      </Glyph>\n      <Item2Launch>\n        <Type>To Common Doc Dir</Type>\n        <Path>Custom Devices\\FPGA Addon\\Windows\\FPGA Addon Configuration.lvlibp\\Addon\\Addon System Explorer\\Main Page.vi</Path>\n      </Item2Launch>\n      <RunTimeMenu>\n        <MenuItem>\n          <GUID>01e8f077-156a-4698-bbdc-a047cf741b9d</GUID>\n          <Type>Action</Type>\n          <Name>\n            <eng>Enable</eng>\n            <loc>Enable</loc>\n          </Name>\n          <Item2Launch>\n            <Type>To Common Doc Dir</Type>\n            <Path>Custom Devices\\FPGA Addon\\Windows\\FPGA Addon Configuration.lvlibp\\Addon\\Addon System Explorer\\RTMs\\EnableDisable Main Page.vi</Path>\n          </Item2Launch>\n        </MenuItem>\n        <MenuItem>\n          <GUID>b2ce9074-10ee-4035-b1de-8d57db17ae03</GUID>\n          <Type>Action</Type>\n          <Name>\n            <eng>Export Config</eng>\n            <loc>Export Config</loc>\n          </Name>\n          <Item2Launch>\n            <Type>To Common Doc Dir</Type>\n            <Path>Custom Devices\\FPGA Addon\\Windows\\FPGA Addon Configuration.lvlibp\\Addon\\Addon System Explorer\\RTMs\\ExportConfigurationToFile.vi</Path>\n          </Item2Launch>\n        </MenuItem>\n        <MenuItem>\n          <GUID>7755077A-1485-13A6-5674A23FB86277FF</GUID>\n          <Type>Separator</Type>\n          <Name>\n            <eng>.</eng>\n            <loc>.</loc>\n          </Name>\n          <Item2Launch>\n            <Type>Absolute</Type>\n            <Path>.</Path>\n          </Item2Launch>\n        </MenuItem>\n        <MenuItem>\n          <GUID>77550670-1485-13A6-568B9AB41979630D</GUID>\n          <Type>Action</Type>\n          <Name>\n            <eng>Delete</eng>\n            <loc>Delete</loc>\n          </Name>\n          <Item2Launch>\n            <Type>Absolute</Type>\n            <Path>Actions\\Delete.vi</Path>\n          </Item2Launch>\n        </MenuItem>\n      </RunTimeMenu>\n      <ActionVIOnLoad>\n        <Type>To Common Doc Dir</Type>\n        <Path>Custom Devices\\FPGA Addon\\Windows\\FPGA Addon Configuration.lvlibp\\Addon\\Addon System Explorer\\Actions\\ActionVIOnLoad.vi</Path>\n      </ActionVIOnLoad>\n    </Page>\n    <Page>\n      <Name>\n        <eng>Scalars</eng>\n        <loc>Scalars</loc>\n      </Name>\n      <DisallowRenaming>true</DisallowRenaming>\n      <DeleteProtection>true</DeleteProtection>\n      <GUID>884b7050-623e-4f2c-925b-6b753ddf9d1a</GUID>\n      <Glyph>\n\t\t  \t<Type>To Application Data Dir</Type>\n\t\t\t  <Path>System Explorer\\Glyphs\\default fpga channel.png</Path>\n\t\t  </Glyph>\n      <Item2Launch>\n        <Type>To Common Doc Dir</Type>\n\t\t    <Path>Custom Devices\\FPGA Addon\\Windows\\FPGA Addon Configuration.lvlibp\\Addon\\Addon System Explorer\\Extra Pages\\Scalars.vi</Path>\n      </Item2Launch>\n      <RunTimeMenu>\n        <MenuItem>\n          <GUID>03D3BE0A-1485-13A6-563AEB9BF271825A</GUID>\n          <Type>VI</Type>\n          <MinNrOfChilds>1</MinNrOfChilds>\n          <Name>\n            <eng>Delete Multiple Items</eng>\n            <loc>Delete Multiple Items</loc>\n          </Name>\n          <Item2Launch>\n            <Type>Absolute</Type>\n            <Path>Dialogs\\Delete Multiple Items.vi</Path>\n          </Item2Launch>\n        </MenuItem>    \n      </RunTimeMenu>\n    </Page>\n    <Page>\n      <Name>\n        <eng>Scalar Inputs</eng>\n        <loc>Scalar Inputs</loc>\n      </Name>\n      <DisallowRenaming>true</DisallowRenaming>\n      <DeleteProtection>true</DeleteProtection>\n      <GUID>45f50bc5-dab3-4e15-b99b-0f8c8c0fe0f0</GUID>\n      <Glyph>\n\t\t  \t<Type>To Application Data Dir</Type>\n\t\t  \t<Path>System Explorer\\Glyphs\\ChnGroup.png</Path>\n\t\t  </Glyph>\n      <Item2Launch>\n        <Type>To Common Doc Dir</Type>\n\t\t    <Path>Custom Devices\\FPGA Addon\\Windows\\FPGA Addon Configuration.lvlibp\\Addon\\Addon System Explorer\\Extra Pages\\Scalar Inputs.vi</Path>\n      </Item2Launch>\n    </Page>\n    <Page>\n      <Name>\n        <eng>Group Input</eng>\n        <loc>Group Input</loc>\n      </Name>\n      <GUID>88748f7d-ce11-4328-8f35-56fd574a40c1</GUID>\n      <Glyph>\n        <Type>To Common Doc Dir</Type>\n\t\t    <Path>Custom Devices\\FPGA Addon\\Windows\\Glyphs\\Group.png</Path>\n\t\t  </Glyph>\n      <Item2Launch>\n        <Type>To Common Doc Dir</Type>\n\t\t    <Path>Custom Devices\\FPGA Addon\\Windows\\FPGA Addon Configuration.lvlibp\\Addon\\Addon System Explorer\\Extra Pages\\Scalar Inputs.vi</Path>\n      </Item2Launch>\n    </Page>\n    <Page>\n      <Name>\n        <eng>Scalar Outputs</eng>\n        <loc>Scalar Outputs</loc>\n      </Name>\n      <DisallowRenaming>true</DisallowRenaming>\n      <DeleteProtection>true</DeleteProtection>\n      <GUID>7d46fed9-731a-4423-8f13-aa8ac2cd791c</GUID>\n      <Glyph>\n\t\t\t  <Type>To Application Data Dir</Type>\n\t\t\t  <Path>System Explorer\\Glyphs\\ChnGroup.png</Path>\n\t\t  </Glyph>\n      <Item2Launch>\n        <Type>To Common Doc Dir</Type>\n\t\t    <Path>Custom Devices\\FPGA Addon\\Windows\\FPGA Addon Configuration.lvlibp\\Addon\\Addon System Explorer\\Extra Pages\\Scalar Outputs.vi</Path>\n      </Item2Launch>\n    </Page>\n    <Page>\n      <Name>\n        <eng>Group Output</eng>\n        <loc>Group Output</loc>\n      </Name>\n      <GUID>58901a15-a42e-477a-af06-3ceeb84f52de</GUID>\n      <Glyph>\n        <Type>To Common Doc Dir</Type>\n\t\t    <Path>Custom Devices\\FPGA Addon\\Windows\\Glyphs\\Group.png</Path>\n\t\t  </Glyph>\n      <Item2Launch>\n        <Type>To Common Doc Dir</Type>\n\t\t    <Path>Custom Devices\\FPGA Addon\\Windows\\FPGA Addon Configuration.lvlibp\\Addon\\Addon System Explorer\\Extra Pages\\Scalar Outputs.vi</Path>\n      </Item2Launch>\n    </Page>\n    <Page>\n      <Name>\n        <eng>Waveforms</eng>\n        <loc>Waveforms</loc>\n      </Name>\n      <DisallowRenaming>true</DisallowRenaming>\n      <DeleteProtection>true</DeleteProtection>\n      <GUID>5f75895a-bfdb-4cd8-9ef2-787e261eba38</GUID>\n      <Glyph>\n\t\t\t  <Type>To Application Data Dir</Type>\n\t\t\t  <Path>System Explorer\\Glyphs\\waveform.png</Path>\n\t\t  </Glyph>\n      <Item2Launch>\n        <Type>To Common Doc Dir</Type>\n\t\t    <Path>Custom Devices\\FPGA Addon\\Windows\\FPGA Addon Configuration.lvlibp\\Addon\\Addon System Explorer\\Extra Pages\\Waveforms.vi</Path>\n      </Item2Launch>\n      <RunTimeMenu>\n        <MenuItem>\n          <GUID>03D3BE0A-1485-13A6-563AEB9BF271825A</GUID>\n          <Type>VI</Type>\n          <MinNrOfChilds>1</MinNrOfChilds>\n          <Name>\n            <eng>Delete Multiple Items</eng>\n            <loc>Delete Multiple Items</loc>\n          </Name>\n          <Item2Launch>\n            <Type>Absolute</Type>\n            <Path>Dialogs\\Delete Multiple Items.vi</Path>\n          </Item2Launch>\n        </MenuItem>\n      </RunTimeMenu>\n    </Page>\n    <Page>\n      <Name>\n        <eng>Waveform Inputs</eng>\n        <loc>Waveform Inputs</loc>\n      </Name>\n      <DisallowRenaming>true</DisallowRenaming>\n      <DeleteProtection>true</DeleteProtection>\n      <ExcludeFromAlphabeticalOrder>true</ExcludeFromAlphabeticalOrder>\n      <GUID>165959cb-b691-43bd-9f8b-54fe62f4b534</GUID>\n      <Glyph>\n\t\t\t  <Type>To Application Data Dir</Type>\n\t\t\t  <Path>System Explorer\\Glyphs\\ChnGroup.png</Path>\n\t\t  </Glyph>\n      <Item2Launch>\n        <Type>To Common Doc Dir</Type>\n\t\t    <Path>Custom Devices\\FPGA Addon\\Windows\\FPGA Addon Configuration.lvlibp\\Addon\\Addon System Explorer\\Extra Pages\\Waveform Inputs.vi</Path>\n      </Item2Launch>\n    </Page>\n    <Page>\n      <Name>\n        <eng>Waveform Outputs</eng>\n        <loc>Waveform Outputs</loc>\n      </Name>\n      <DisallowRenaming>true</DisallowRenaming>\n      <DeleteProtection>true</DeleteProtection>\n      <ExcludeFromAlphabeticalOrder>true</ExcludeFromAlphabeticalOrder>\n      <GUID>bc66db3e-ace6-4d58-add4-89e89e885df7</GUID>\n      <Glyph>\n        <Type>To Application Data Dir</Type>\n        <Path>System Explorer\\Glyphs\\ChnGroup.png</Path>\n      </Glyph>\n      <Item2Launch>\n        <Type>To Common Doc Dir</Type>\n        <Path>Custom Devices\\FPGA Addon\\Windows\\FPGA Addon Configuration.lvlibp\\Addon\\Addon System Explorer\\Extra Pages\\Waveform Outputs.vi</Path>\n      </Item2Launch>\n    </Page>\n    <Page>\n      <Name>\n        <eng>Scalar Input</eng>\n        <loc>Scalar Input</loc>\n      </Name>\n      <GUID>9bd0c044-925c-4d1d-a44e-de3c4043858c</GUID>\n      <Glyph>\n\t\t  \t<Type>To Application Data Dir</Type>\n\t\t  \t<Path>System Explorer\\Glyphs\\default fpga channel.png</Path>\n\t\t  </Glyph>\n      <Item2Launch>\n        <Type>To Common Doc Dir</Type>\n\t\t    <Path>Custom Devices\\FPGA Addon\\Windows\\FPGA Addon Configuration.lvlibp\\Addon\\Addon System Explorer\\Extra Pages\\Scalar Input.vi</Path>\n      </Item2Launch>\n      <RunTimeMenu>\n        <MenuItem>\n          <GUID>2cd33a82-ccc0-4cb3-affc-1385b5dc0dd8</GUID>\n          <Type>Action</Type>\n          <Name>\n            <eng>Enable Bitpacked</eng>\n            <loc>Enable Bitpacked</loc>\n          </Name>\n          <Item2Launch>\n            <Type>To Common Doc Dir</Type>\n            <Path>Custom Devices\\FPGA Addon\\Windows\\FPGA Addon Configuration.lvlibp\\Addon\\Addon System Explorer\\RTMs\\Switch Scalar Type.vi</Path>\n          </Item2Launch>\n        </MenuItem>\n        <MenuItem>\n          <GUID>7755077A-1485-13A6-5674A23FB86277FF</GUID>\n          <Type>Separator</Type>\n          <Name>\n            <eng>.</eng>\n            <loc>.</loc>\n          </Name>\n          <Item2Launch>\n            <Type>Absolute</Type>\n            <Path>.</Path>\n          </Item2Launch>\n        </MenuItem>\n        <MenuItem>\n          <GUID>77550670-1485-13A6-568B9AB41979630D</GUID>\n          <Type>Action</Type>\n          <Name>\n            <eng>Delete</eng>\n            <loc>Delete</loc>\n          </Name>\n          <Item2Launch>\n            <Type>Absolute</Type>\n            <Path>Actions\\Delete.vi</Path>\n          </Item2Launch>\n        </MenuItem>\n      </RunTimeMenu>\n    </Page>\n    <Page>\n      <Name>\n        <eng>Scalar Output</eng>\n        <loc>Scalar Output</loc>\n      </Name>\n      <GUID>625afbbf-e929-46eb-93d1-fe7033ba1e7b</GUID>\n      <Glyph>\n\t\t  \t<Type>To Application Data Dir</Type>\n\t\t  \t<Path>System Explorer\\Glyphs\\default fpga channel.png</Path>\n\t  \t</Glyph>\n      <Item2Launch>\n        <Type>To Common Doc Dir</Type>\n\t\t    <Path>Custom Devices\\FPGA Addon\\Windows\\FPGA Addon Configuration.lvlibp\\Addon\\Addon System Explorer\\Extra Pages\\Scalar Output.vi</Path>\n      </Item2Launch>\n      <RunTimeMenu>\n        <MenuItem>\n          <GUID>2cd33a82-ccc0-4cb3-affc-1385b5dc0dd8</GUID>\n          <Type>Action</Type>\n          <Name>\n            <eng>Enable Bitpacked</eng>\n            <loc>Enable Bitpacked</loc>\n          </Name>\n          <Item2Launch>\n            <Type>To Common Doc Dir</Type>\n            <Path>Custom Devices\\FPGA Addon\\Windows\\FPGA Addon Configuration.lvlibp\\Addon\\Addon System Explorer\\RTMs\\Switch Scalar Type.vi</Path>\n          </Item2Launch>\n        </MenuItem>\n        <MenuItem>\n          <GUID>7755077A-1485-13A6-5674A23FB86277FF</GUID>\n          <Type>Separator</Type>\n          <Name>\n            <eng>.</eng>\n            <loc>.</loc>\n          </Name>\n          <Item2Launch>\n            <Type>Absolute</Type>\n            <Path>.</Path>\n          </Item2Launch>\n        </MenuItem>\n        <MenuItem>\n          <GUID>77550670-1485-13A6-568B9AB41979630D</GUID>\n          <Type>Action</Type>\n          <Name>\n            <eng>Delete</eng>\n            <loc>Delete</loc>\n          </Name>\n          <Item2Launch>\n            <Type>Absolute</Type>\n            <Path>Actions\\Delete.vi</Path>\n          </Item2Launch>\n        </MenuItem>\n      </RunTimeMenu>\n    </Page>\n    <Page>\n      <Name>\n        <eng>DMA</eng>\n        <loc>DMA</loc>\n      </Name>\n      <ExcludeFromAlphabeticalOrder>true</ExcludeFromAlphabeticalOrder>\n      <GUID>fdfaa619-d09f-452b-8143-c1a261c13b7a</GUID>\n      <Glyph>\n\t\t\t  <Type>To Application Data Dir</Type>\n\t\t\t  <Path>System Explorer\\Glyphs\\Lookup Table.png</Path>\n\t\t  </Glyph>\n      <Item2Launch>\n        <Type>To Common Doc Dir</Type>\n\t\t    <Path>Custom Devices\\FPGA Addon\\Windows\\FPGA Addon Configuration.lvlibp\\Addon\\Addon System Explorer\\Extra Pages\\DMA Channel.vi</Path>\n      </Item2Launch>\n      <RunTimeMenu>\n         <MenuItem>\n            <GUID>345ad323-e622-4d27-9f97-b3d588c29827</GUID>\n            <Type>Action</Type>\n            <Name>\n              <eng>Import DMA Channels</eng>\n              <loc>Import DMA Channels</loc>\n            </Name>\n            <Item2Launch>\n              <Type>To Common Doc Dir</Type>\n              <Path>Custom Devices\\FPGA Addon\\Windows\\FPGA Addon Configuration.lvlibp\\Addon\\Addon System Explorer\\RTMs\\Import DMA Channels RTM.vi</Path>\n            </Item2Launch>\n          </MenuItem>\n          <MenuItem>\n            <GUID>7755077A-1485-13A6-5674A23FB86277FF</GUID>\n            <Type>Separator</Type>\n            <Name>\n              <eng>.</eng>\n              <loc>.</loc>\n            </Name>\n            <Item2Launch>\n              <Type>Absolute</Type>\n              <Path>.</Path>\n            </Item2Launch>\n          </MenuItem>\n      </RunTimeMenu>\n    <ButtonList>\n        <Button>\n          <ID>Import DMA Channels</ID>\n          <Glyph>\n            <Type>To Application Data Dir</Type>\n            <Path>System Explorer\\Glyphs\\NI-XNET ImportXNETFrames.png</Path>\n          </Glyph>\n          <Type>Action</Type>\n          <ReferencedGUID>345ad323-e622-4d27-9f97-b3d588c29827</ReferencedGUID>\n          <ButtonText>\n            <eng>Import DMA Channels</eng>\n            <loc>Import DMA Channels</loc>\n          </ButtonText>\n          <Caption>\n            <eng>Import DMA Channels</eng>\n            <loc>Import DMA Channels</loc>\n          </Caption>\n          <TipStrip>\n            <eng>Import DMA Channels</eng>\n            <loc>Import DMA Channels</loc>\n          </TipStrip>\n          <Documentation>\n            <eng/>\n            <loc/>\n          </Documentation>\n        </Button>\n    </ButtonList>\n    </Page>\n    <Page>\n      <Name>\n        <eng>Waveform Output</eng>\n        <loc>Waveform Output</loc>\n      </Name>\n      <DeleteProtection>true</DeleteProtection>\n      <ExcludeFromAlphabeticalOrder>true</ExcludeFromAlphabeticalOrder>\n      <GUID>0c0ecc88-7768-47db-a589-856e32a93156</GUID>\n      <Glyph>\n        <Type>To Application Data Dir</Type>\n        <Path>System Explorer\\Glyphs\\waveform.png</Path>\n      </Glyph>\n      <Item2Launch>\n        <Type>To Common Doc Dir</Type>\n        <Path>Custom Devices\\FPGA Addon\\Windows\\FPGA Addon Configuration.lvlibp\\Addon\\Addon System Explorer\\Extra Pages\\Waveform Output.vi</Path>\n      </Item2Launch>\n    </Page>\n    <Page>\n      <Name>\n        <eng>Waveform Input</eng>\n        <loc>Waveform Input</loc>\n      </Name>\n      <DeleteProtection>true</DeleteProtection>\n      <ExcludeFromAlphabeticalOrder>true</ExcludeFromAlphabeticalOrder>\n      <GUID>2afc1de4-b056-47bb-a2ad-eec5ad0d30b6</GUID>\n      <Glyph>\n        <Type>To Application Data Dir</Type>\n        <Path>System Explorer\\Glyphs\\waveform.png</Path>\n      </Glyph>\n      <Item2Launch>\n        <Type>To Common Doc Dir</Type>\n        <Path>Custom Devices\\FPGA Addon\\Windows\\FPGA Addon Configuration.lvlibp\\Addon\\Addon System Explorer\\Extra Pages\\Waveform Input.vi</Path>\n      </Item2Launch>\n    </Page>\n    <Page>\n      <Name>\n        <eng>DMA Status Channels</eng>\n        <loc>DMA Status Channels</loc>\n      </Name>\n      <DisallowRenaming>true</DisallowRenaming>\n      <DeleteProtection>true</DeleteProtection>\n      <ExcludeFromAlphabeticalOrder>true</ExcludeFromAlphabeticalOrder>\n      <GUID>4e1a084b-2b8b-4128-8417-f0007d9ffe93</GUID>\n      <Glyph>\n\t\t  \t<Type>To Application Data Dir</Type>\n\t\t  \t<Path>System Explorer\\Glyphs\\event-based.png</Path>\n\t\t  </Glyph>\n      <Item2Launch>\n        <Type>To Common Doc Dir</Type>\n\t    \t<Path>Custom Devices\\FPGA Addon\\Windows\\FPGA Addon Configuration.lvlibp\\Addon\\Addon System Explorer\\Extra Pages\\DMA Status Channels.vi</Path>\n      </Item2Launch>\n    </Page>\n    <Page>\n      <Name>\n        <eng>DMA Error</eng>\n        <loc>DMA Error</loc>\n      </Name>\n      <DisallowRenaming>true</DisallowRenaming>\n      <DeleteProtection>true</DeleteProtection>\n      <GUID>708ff167-b4eb-405e-bb0f-5c2fb305da21</GUID>\n      <Glyph>\n        <Type>To Application Data Dir</Type>\n        <Path>System Explorer\\Glyphs\\RM Information Channels.png</Path>\n      </Glyph>\n      <Item2Launch>\n        <Type>To Common Doc Dir</Type>\n        <Path>Custom Devices\\FPGA Addon\\Windows\\FPGA Addon Configuration.lvlibp\\Addon\\Addon System Explorer\\Extra Pages\\DMA Error.vi</Path>\n      </Item2Launch>\n    </Page>\n    <Page>\n      <Name>\n        <eng>DMA Elements Remaining</eng>\n        <loc>DMA Elements Remaining</loc>\n      </Name>\n      <DisallowRenaming>true</DisallowRenaming>\n      <DeleteProtection>true</DeleteProtection>\n      <GUID>785497d1-fc1e-46c9-8feb-aa61f2850cff</GUID>\n      <Glyph>\n        <Type>To Application Data Dir</Type>\n        <Path>System Explorer\\Glyphs\\RM Information Channels.png</Path>\n      </Glyph>\n      <Item2Launch>\n        <Type>To Common Doc Dir</Type>\n        <Path>Custom Devices\\FPGA Addon\\Windows\\FPGA Addon Configuration.lvlibp\\Addon\\Addon System Explorer\\Extra Pages\\DMA Elements Remaining.vi</Path>\n      </Item2Launch>\n    </Page>\n    <Page>\n      <Name>\n        <eng>Scalar Input Bitpacked</eng>\n        <loc>Scalar Input Bitpacked</loc>\n      </Name>\n      <ExcludeFromAlphabeticalOrder>true</ExcludeFromAlphabeticalOrder>\n      <GUID>8489bf21-57e3-4e68-bdd5-eadff573ec1e</GUID>\n      <Glyph>\n        <Type>To Common Doc Dir</Type>\n\t\t  <Path>Custom Devices\\FPGA Addon\\Windows\\Glyphs\\Bitpacked.png</Path>\n      </Glyph>\n      <Item2Launch>\n        <Type>To Common Doc Dir</Type>\n        <Path>Custom Devices\\FPGA Addon\\Windows\\FPGA Addon Configuration.lvlibp\\Addon\\Addon System Explorer\\Extra Pages\\Scalar Bitpacked.vi</Path>\n      </Item2Launch>\n      <RunTimeMenu>\n        <MenuItem>\n          <GUID>2cd33a82-ccc0-4cb3-affc-1385b5dc0dd8</GUID>\n          <Type>Action</Type>\n          <Name>\n            <eng>Disable Bitpacked</eng>\n            <loc>Disable Bitpacked</loc>\n          </Name>\n          <Item2Launch>\n            <Type>To Common Doc Dir</Type>\n            <Path>Custom Devices\\FPGA Addon\\Windows\\FPGA Addon Configuration.lvlibp\\Addon\\Addon System Explorer\\RTMs\\Switch Scalar Type.vi</Path>\n          </Item2Launch>\n        </MenuItem>\n        <MenuItem>\n          <GUID>7755077A-1485-13A6-5674A23FB86277FF</GUID>\n          <Type>Separator</Type>\n          <Name>\n            <eng>.</eng>\n            <loc>.</loc>\n          </Name>\n          <Item2Launch>\n            <Type>Absolute</Type>\n            <Path>.</Path>\n          </Item2Launch>\n        </MenuItem>\n        <MenuItem>\n          <GUID>77550670-1485-13A6-568B9AB41979630D</GUID>\n          <Type>Action</Type>\n          <Name>\n            <eng>Delete</eng>\n            <loc>Delete</loc>\n          </Name>\n          <Item2Launch>\n            <Type>Absolute</Type>\n            <Path>Actions\\Delete.vi</Path>\n          </Item2Launch>\n        </MenuItem>\n      </RunTimeMenu>\n    </Page>\n    <Page>\n      <Name>\n        <eng>Scalar Output Bitpacked</eng>\n        <loc>Scalar Output Bitpacked</loc>\n      </Name>\n      <ExcludeFromAlphabeticalOrder>true</ExcludeFromAlphabeticalOrder>\n      <GUID>ebfc3e29-7579-49df-b828-0da2c3787b5f</GUID>\n      <Glyph>\n        <Type>To Common Doc Dir</Type>\n\t\t  <Path>Custom Devices\\FPGA Addon\\Windows\\Glyphs\\Bitpacked.png</Path>\n      </Glyph>\n      <Item2Launch>\n        <Type>To Common Doc Dir</Type>\n        <Path>Custom Devices\\FPGA Addon\\Windows\\FPGA Addon Configuration.lvlibp\\Addon\\Addon System Explorer\\Extra Pages\\Scalar Bitpacked.vi</Path>\n      </Item2Launch>\n      <RunTimeMenu>\n        <MenuItem>\n          <GUID>2cd33a82-ccc0-4cb3-affc-1385b5dc0dd8</GUID>\n          <Type>Action</Type>\n          <Name>\n            <eng>Disable Bitpacked</eng>\n            <loc>Disable Bitpacked</loc>\n          </Name>\n          <Item2Launch>\n            <Type>To Common Doc Dir</Type>\n            <Path>Custom Devices\\FPGA Addon\\Windows\\FPGA Addon Configuration.lvlibp\\Addon\\Addon System Explorer\\RTMs\\Switch Scalar Type.vi</Path>\n          </Item2Launch>\n        </MenuItem>\n        <MenuItem>\n          <GUID>7755077A-1485-13A6-5674A23FB86277FF</GUID>\n          <Type>Separator</Type>\n          <Name>\n            <eng>.</eng>\n            <loc>.</loc>\n          </Name>\n          <Item2Launch>\n            <Type>Absolute</Type>\n            <Path>.</Path>\n          </Item2Launch>\n        </MenuItem>\n        <MenuItem>\n          <GUID>77550670-1485-13A6-568B9AB41979630D</GUID>\n          <Type>Action</Type>\n          <Name>\n            <eng>Delete</eng>\n            <loc>Delete</loc>\n          </Name>\n          <Item2Launch>\n            <Type>Absolute</Type>\n            <Path>Actions\\Delete.vi</Path>\n          </Item2Launch>\n        </MenuItem>\n      </RunTimeMenu>\n    </Page>\n    <Page>\n      <Name>\n        <eng>Bitpacked Input</eng>\n        <loc>Bitpacked Input</loc>\n      </Name>\n      <DeleteProtection>true</DeleteProtection>\n      <ExcludeFromAlphabeticalOrder>true</ExcludeFromAlphabeticalOrder>\n      <GUID>4b03cffd-e469-431a-ba96-aca85ece66af</GUID>\n      <Glyph>\n        <Type>To Application Data Dir</Type>\n        <Path>System Explorer\\Glyphs\\default fpga channel.png</Path>\n      </Glyph>\n      <Item2Launch>\n        <Type>To Common Doc Dir</Type>\n        <Path>Custom Devices\\FPGA Addon\\Windows\\FPGA Addon Configuration.lvlibp\\Addon\\Addon System Explorer\\Extra Pages\\Scalar Input.vi</Path>\n      </Item2Launch>\n    </Page>\n    <Page>\n      <Name>\n        <eng>Bitpacked Output</eng>\n        <loc>Bitpacked Output</loc>\n      </Name>\n      <DeleteProtection>true</DeleteProtection>\n      <ExcludeFromAlphabeticalOrder>true</ExcludeFromAlphabeticalOrder>\n      <GUID>6db3f02b-654f-4ed6-bd84-80bb5242a557</GUID>\n      <Glyph>\n        <Type>To Application Data Dir</Type>\n        <Path>System Explorer\\Glyphs\\default fpga channel.png</Path>\n      </Glyph>\n      <Item2Launch>\n        <Type>To Common Doc Dir</Type>\n        <Path>Custom Devices\\FPGA Addon\\Windows\\FPGA Addon Configuration.lvlibp\\Addon\\Addon System Explorer\\Extra Pages\\Scalar Output.vi</Path>\n      </Item2Launch>\n    </Page>\n      <Page>\n      <Name>\n        <eng>Static Scalar Input</eng>\n        <loc>Static Scalar Input</loc>\n      </Name>\n      <GUID>7579cb69-d559-4b2b-a1fc-0d112e8661b6</GUID>\n      <Glyph>\n        <Type>To Application Data Dir</Type>\n        <Path>System Explorer\\Glyphs\\default fpga channel.png</Path>\n      </Glyph>\n      <Item2Launch>\n        <Type>To Common Doc Dir</Type>\n        <Path>Custom Devices\\FPGA Addon\\Windows\\FPGA Addon Configuration.lvlibp\\Addon\\Addon System Explorer\\Extra Pages\\Scalar Input.vi</Path>\n      </Item2Launch>\n      <RunTimeMenu>\n        <MenuItem>\n          <GUID>77550670-1485-13A6-568B9AB41979630D</GUID>\n          <Type>Action</Type>\n          <Name>\n            <eng>Delete</eng>\n            <loc>Delete</loc>\n          </Name>\n          <Item2Launch>\n            <Type>Absolute</Type>\n            <Path>Actions\\Delete.vi</Path>\n          </Item2Launch>\n        </MenuItem>\n      </RunTimeMenu>\n    </Page>\n    <Page>\n      <Name>\n        <eng>Static Scalar Output</eng>\n        <loc>Static Scalar Output</loc>\n      </Name>\n      <GUID>ddc5186b-4b14-4629-b48a-cef4575f789c</GUID>\n      <Glyph>\n        <Type>To Application Data Dir</Type>\n        <Path>System Explorer\\Glyphs\\default fpga channel.png</Path>\n      </Glyph>\n      <Item2Launch>\n        <Type>To Common Doc Dir</Type>\n        <Path>Custom Devices\\FPGA Addon\\Windows\\FPGA Addon Configuration.lvlibp\\Addon\\Addon System Explorer\\Extra Pages\\Scalar Output.vi</Path>\n      </Item2Launch>\n      <RunTimeMenu>\n        <MenuItem>\n          <GUID>77550670-1485-13A6-568B9AB41979630D</GUID>\n          <Type>Action</Type>\n          <Name>\n            <eng>Delete</eng>\n            <loc>Delete</loc>\n          </Name>\n          <Item2Launch>\n            <Type>Absolute</Type>\n            <Path>Actions\\Delete.vi</Path>\n          </Item2Launch>\n        </MenuItem>\n      </RunTimeMenu>\n    </Page>\n      <Page>\n      <Name>\n        <eng>Speciality IO</eng>\n        <loc>Speciality IO</loc>\n      </Name>\n      <ExcludeFromAlphabeticalOrder>true</ExcludeFromAlphabeticalOrder>\n      <GUID>25832021-24b6-475a-aa84-f4ed7870ed99</GUID>\n      <Glyph>\n        <Type>To Common Doc Dir</Type>\n\t\t  <Path>Custom Devices\\FPGA Addon\\Windows\\Glyphs\\IP Core.png</Path>\n      </Glyph>\n      <Item2Launch>\n        <Type>To Common Doc Dir</Type>\n        <Path>Custom Devices\\FPGA Addon\\Windows\\FPGA Addon Configuration.lvlibp\\Addon\\Addon System Explorer\\Extra Pages\\Speciality IO.vi</Path>\n      </Item2Launch>\n    </Page>\n  </Pages>\n  <CustomXML>\n    <Dummy/>\n  </CustomXML>\n</CustomDevice>", "<?xml version=\"1.0\" encoding=\"utf-8\" standalone=\"no\" ?><CustomDevice xmlns:xsi=\"http://www.w3.org/2001/XMLSchema-instance\" xsi:noNamespaceSchemaLocation=\"Custom Device.xsd\">\n<XSDVersion Build=\"0\" Fix=\"0\" Major=\"2010\" Minor=\"0\"/>\n  <AddMenu>\n    <eng>NI::FPGA Addon</eng>\n    <loc>NI::FPGA Addon</loc>\n  </AddMenu>\n  <Version>3.3.1</Version>\n  <Type>Inline HW Interface</Type>\n  <MaxOccurrence>-1</MaxOccurrence>\n  <MainPageGUID>e80a28c5-621d-4211-b584-b71df509dee0</MainPageGUID>\n  <InitializationVI>\n    <Type>Action</Type>\n    <Item2Launch>\n      <Type>To Common Doc Dir</Type>\n\t\t<Path>Custom Devices\\FPGA Addon\\Windows\\FPGA Addon Configuration.lvlibp\\Addon\\Addon System Explorer\\Initialization VI.vi</Path>\n    </Item2Launch>\n  </InitializationVI>\n  <CustomDeviceVI>\n\t<SourceDistribution>\n\t\t<Source>\n\t\t\t<SupportedTarget>Windows</SupportedTarget>\n\t\t\t<Source>\n\t\t\t\t<Type>To Common Doc Dir</Type>\n\t\t\t\t<Path>Custom Devices\\FPGA Addon\\Windows\\FPGA Addon Engine Windows.lvlibp\\Addon\\Addon Engine\\RT Driver VI.vi</Path>\n\t\t\t</Source>\n\t\t\t<RealTimeSystemDestination>c:\\ni-rt\\VeriStand\\Custom Devices\\FPGA Addon\\FPGA Addon Engine Windows.lvlibp\\Addon\\Addon Engine\\RT Driver VI.vi</RealTimeSystemDestination>\n\t\t</Source>\n\t\t<Source>\n\t\t\t<SupportedTarget>Linux_x64</SupportedTarget>\n\t\t\t<Source>\n\t\t\t\t<Type>To Common Doc Dir</Type>\n\t\t\t\t<Path>Custom Devices\\FPGA Addon\\Linux_x64\\FPGA Addon Engine Linux64.lvlibp\\Addon\\Addon Engine\\RT Driver VI.vi</Path>\n\t\t\t</Source>\n\t\t\t<RealTimeSystemDestination>c:\\ni-rt\\VeriStand\\Custom Devices\\FPGA Addon\\FPGA Addon Engine Linux64.lvlibp\\Addon\\Addon Engine\\RT Driver VI.vi</RealTimeSystemDestination>\n\t\t</Source>\n\t</SourceDistribution>\n\t</CustomDeviceVI>\n  <Dependencies/>\n  <Pages>\n    <Page>\n      <Name>\n        <eng>FPGA Addon</eng>\n        <loc>FPGA Addon</loc>\n      </Name>\n      <GUID>e80a28c5-621d-4211-b584-b71df509dee0</GUID>\n      <Glyph>\n\t\t  \t<Type>To Application Data Dir</Type>\n\t\t\t  <Path>System Explorer\\Glyphs\\fpga device.png</Path>\n\t\t  </Glyph>\n      <Item2Launch>\n        <Type>To Common Doc Dir</Type>\n\t\t    <Path>Custom Devices\\FPGA Addon\\Windows\\FPGA Addon Configuration.lvlibp\\Addon\\Addon System Explorer\\Main Page.vi</Path>\n      </Item2Launch>\n      <RunTimeMenu>\n        <MenuItem>\n          <GUID>01e8f077-156a-4698-bbdc-a047cf741b9d</GUID>\n          <Type>Action</Type>\n          <Name>\n            <eng>Disable</eng>\n            <loc>Disable</loc>\n          </Name>\n          <Item2Launch>\n            <Type>To Common Doc Dir</Type>\n            <Path>Custom Devices\\FPGA Addon\\Windows\\FPGA Addon Configuration.lvlibp\\Addon\\Addon System Explorer\\RTMs\\EnableDisable Main Page.vi</Path>\n          </Item2Launch>\n        </MenuItem>\n        <MenuItem>\n\t\t\t\t\t<GUID>b2ce9074-10ee-4035-b1de-8d57db17ae03</GUID>\n\t\t\t\t\t<Type>Action</Type>\n\t\t\t\t\t<Name>\n\t\t\t\t\t\t<eng>Export Config</eng>\n\t\t\t\t\t\t<loc>Export Config</loc>\n\t\t\t\t\t</Name>\n\t\t\t\t\t<Item2Launch>\n\t\t\t\t\t\t<Type>To Common Doc Dir</Type>\n\t\t\t\t\t\t<Path>Custom Devices\\FPGA Addon\\Windows\\FPGA Addon Configuration.lvlibp\\Addon\\Addon System Explorer\\RTMs\\ExportConfigurationToFile.vi</Path>\n\t\t\t\t\t</Item2Launch>\n\t\t\t\t</MenuItem>\n        <MenuItem>\n          <GUID>7755077A-1485-13A6-5674A23FB86277FF</GUID>\n          <Type>Separator</Type>\n          <Name>\n            <eng>.</eng>\n            <loc>.</loc>\n          </Name>\n          <Item2Launch>\n            <Type>Absolute</Type>\n            <Path>.</Path>\n          </Item2Launch>\n        </MenuItem>\n        <MenuItem>\n          <GUID>77550670-1485-13A6-568B9AB41979630D</GUID>\n          <Type>Action</Type>\n          <Name>\n            <eng>Delete</eng>\n            <loc>Delete</loc>\n          </Name>\n          <Item2Launch>\n            <Type>Absolute</Type>\n            <Path>Actions\\Delete.vi</Path>\n          </Item2Launch>\n        </MenuItem>\n      </RunTimeMenu>\n      <ActionVIOnLoad>\n        <Type>To Common Doc Dir</Type>\n        <Path>Custom Devices\\FPGA Addon\\Windows\\FPGA Addon Configuration.lvlibp\\Addon\\Addon System Explorer\\Actions\\ActionVIOnLoad.vi</Path>\n      </ActionVIOnLoad>\n      <ActionVIOnCompile>\n        <Type>To Common Doc Dir</Type>\n        <Path>Custom Devices\\FPGA Addon\\Windows\\FPGA Addon Configuration.lvlibp\\Addon\\Addon System Explorer\\Actions\\ActionVIOnCompile.vi</Path>\n      </ActionVIOnCompile>\n    </Page>\n    <Page>\n      <Name>\n        <eng>FPGA Addon</eng>\n        <loc>FPGA Addon</loc>\n      </Name>\n      <GUID>1903f8c0-e426-4f25-b8ca-65973b1160fd</GUID>\n      <Glyph>\n        <Type>To Application Data Dir</Type>\n        <Path>System Explorer\\Glyphs\\fpga device_disabled.png</Path>\n      </Glyph>\n      <Item2Launch>\n        <Type>To Common Doc Dir</Type>\n        <Path>Custom Devices\\FPGA Addon\\Windows\\FPGA Addon Configuration.lvlibp\\Addon\\Addon System Explorer\\Main Page.vi</Path>\n      </Item2Launch>\n      <RunTimeMenu>\n        <MenuItem>\n          <GUID>01e8f077-156a-4698-bbdc-a047cf741b9d</GUID>\n          <Type>Action</Type>\n          <Name>\n            <eng>Enable</eng>\n            <loc>Enable</loc>\n          </Name>\n          <Item2Launch>\n            <Type>To Common Doc Dir</Type>\n            <Path>Custom Devices\\FPGA Addon\\Windows\\FPGA Addon Configuration.lvlibp\\Addon\\Addon System Explorer\\RTMs\\EnableDisable Main Page.vi</Path>\n          </Item2Launch>\n        </MenuItem>\n        <MenuItem>\n          <GUID>b2ce9074-10ee-4035-b1de-8d57db17ae03</GUID>\n          <Type>Action</Type>\n          <Name>\n            <eng>Export Config</eng>\n            <loc>Export Config</loc>\n          </Name>\n          <Item2Launch>\n            <Type>To Common Doc Dir</Type>\n            <Path>Custom Devices\\FPGA Addon\\Windows\\FPGA Addon Configuration.lvlibp\\Addon\\Addon System Explorer\\RTMs\\ExportConfigurationToFile.vi</Path>\n          </Item2Launch>\n        </MenuItem>\n        <MenuItem>\n          <GUID>7755077A-1485-13A6-5674A23FB86277FF</GUID>\n          <Type>Separator</Type>\n          <Name>\n            <eng>.</eng>\n            <loc>.</loc>\n          </Name>\n          <Item2Launch>\n            <Type>Absolute</Type>\n            <Path>.</Path>\n          </Item2Launch>\n        </MenuItem>\n        <MenuItem>\n          <GUID>77550670-1485-13A6-568B9AB41979630D</GUID>\n          <Type>Action</Type>\n          <Name>\n            <eng>Delete</eng>\n            <loc>Delete</loc>\n          </Name>\n          <Item2Launch>\n            <Type>Absolute</Type>\n            <Path>Actions\\Delete.vi</Path>\n          </Item2Launch>\n        </MenuItem>\n      </RunTimeMenu>\n      <ActionVIOnLoad>\n        <Type>To Common Doc Dir</Type>\n        <Path>Custom Devices\\FPGA Addon\\Windows\\FPGA Addon Configuration.lvlibp\\Addon\\Addon System Explorer\\Actions\\ActionVIOnLoad.vi</Path>\n      </ActionVIOnLoad>\n    </Page>\n    <Page>\n      <Name>\n        <eng>Scalars</eng>\n        <loc>Scalars</loc>\n      </Name>\n      <DisallowRenaming>true</DisallowRenaming>\n      <DeleteProtection>true</DeleteProtection>\n      <GUID>884b7050-623e-4f2c-925b-6b753ddf9d1a</GUID>\n      <Glyph>\n\t\t  \t<Type>To Application Data Dir</Type>\n\t\t\t  <Path>System Explorer\\Glyphs\\default fpga channel.png</Path>\n\t\t  </Glyph>\n      <Item2Launch>\n        <Type>To Common Doc Dir</Type>\n\t\t    <Path>Custom Devices\\FPGA Addon\\Windows\\FPGA Addon Configuration.lvlibp\\Addon\\Addon System Explorer\\Extra Pages\\Scalars.vi</Path>\n      </Item2Launch>\n      <RunTimeMenu>\n        <MenuItem>\n          <GUID>03D3BE0A-1485-13A6-563AEB9BF271825A</GUID>\n          <Type>VI</Type>\n          <MinNrOfChilds>1</MinNrOfChilds>\n          <Name>\n            <eng>Delete Multiple Items</eng>\n            <loc>Delete Multiple Items</loc>\n          </Name>\n          <Item2Launch>\n            <Type>Absolute</Type>\n            <Path>Dialogs\\Delete Multiple Items.vi</Path>\n          </Item2Launch>\n        </MenuItem>    \n      </RunTimeMenu>\n    </Page>\n    <Page>\n      <Name>\n        <eng>Scalar Inputs</eng>\n        <loc>Scalar Inputs</loc>\n      </Name>\n      <DisallowRenaming>true</DisallowRenaming>\n      <DeleteProtection>true</DeleteProtection>\n      <GUID>45f50bc5-dab3-4e15-b99b-0f8c8c0fe0f0</GUID>\n      <Glyph>\n\t\t  \t<Type>To Application Data Dir</Type>\n\t\t  \t<Path>System Explorer\\Glyphs\\ChnGroup.png</Path>\n\t\t  </Glyph>\n      <Item2Launch>\n        <Type>To Common Doc Dir</Type>\n\t\t    <Path>Custom Devices\\FPGA Addon\\Windows\\FPGA Addon Configuration.lvlibp\\Addon\\Addon System Explorer\\Extra Pages\\Scalar Inputs.vi</Path>\n      </Item2Launch>\n    </Page>\n    <Page>\n      <Name>\n        <eng>Group Input</eng>\n        <loc>Group Input</loc>\n      </Name>\n      <GUID>88748f7d-ce11-4328-8f35-56fd574a40c1</GUID>\n      <Glyph>\n        <Type>To Common Doc Dir</Type>\n\t\t    <Path>Custom Devices\\FPGA Addon\\Windows\\Glyphs\\Group.png</Path>\n\t\t  </Glyph>\n      <Item2Launch>\n        <Type>To Common Doc Dir</Type>\n\t\t    <Path>Custom Devices\\FPGA Addon\\Windows\\FPGA Addon Configuration.lvlibp\\Addon\\Addon System Explorer\\Extra Pages\\Scalar Inputs.vi</Path>\n      </Item2Launch>\n    </Page>\n    <Page>\n      <Name>\n        <eng>Scalar Outputs</eng>\n        <loc>Scalar Outputs</loc>\n      </Name>\n      <DisallowRenaming>true</DisallowRenaming>\n      <DeleteProtection>true</DeleteProtection>\n      <GUID>7d46fed9-731a-4423-8f13-aa8ac2cd791c</GUID>\n      <Glyph>\n\t\t\t  <Type>To Application Data Dir</Type>\n\t\t\t  <Path>System Explorer\\Glyphs\\ChnGroup.png</Path>\n\t\t  </Glyph>\n      <Item2Launch>\n        <Type>To Common Doc Dir</Type>\n\t\t    <Path>Custom Devices\\FPGA Addon\\Windows\\FPGA Addon Configuration.lvlibp\\Addon\\Addon System Explorer\\Extra Pages\\Scalar Outputs.vi</Path>\n      </Item2Launch>\n    </Page>\n    <Page>\n      <Name>\n        <eng>Group Output</eng>\n        <loc>Group Output</loc>\n      </Name>\n      <GUID>58901a15-a42e-477a-af06-3ceeb84f52de</GUID>\n      <Glyph>\n        <Type>To Common Doc Dir</Type>\n\t\t    <Path>Custom Devices\\FPGA Addon\\Windows\\Glyphs\\Group.png</Path>\n\t\t  </Glyph>\n      <Item2Launch>\n        <Type>To Common Doc Dir</Type>\n\t\t    <Path>Custom Devices\\FPGA Addon\\Windows\\FPGA Addon Configuration.lvlibp\\Addon\\Addon System Explorer\\Extra Pages\\Scalar Outputs.vi</Path>\n      </Item2Launch>\n    </Page>\n    <Page>\n      <Name>\n        <eng>Waveforms</eng>\n        <loc>Waveforms</loc>\n      </Name>\n      <DisallowRenaming>true</DisallowRenaming>\n      <DeleteProtection>true</DeleteProtection>\n      <GUID>5f75895a-bfdb-4cd8-9ef2-787e261eba38</GUID>\n      <Glyph>\n\t\t\t  <Type>To Application Data Dir</Type>\n\t\t\t  <Path>System Explorer\\Glyphs\\waveform.png</Path>\n\t\t  </Glyph>\n      <Item2Launch>\n        <Type>To Common Doc Dir</Type>\n\t\t    <Path>Custom Devices\\FPGA Addon\\Windows\\FPGA Addon Configuration.lvlibp\\Addon\\Addon System Explorer\\Extra Pages\\Waveforms.vi</Path>\n      </Item2Launch>\n      <RunTimeMenu>\n        <MenuItem>\n          <GUID>03D3BE0A-1485-13A6-563AEB9BF271825A</GUID>\n          <Type>VI</Type>\n          <MinNrOfChilds>1</MinNrOfChilds>\n          <Name>\n            <eng>Delete Multiple Items</eng>\n            <loc>Delete Multiple Items</loc>\n          </Name>\n          <Item2Launch>\n            <Type>Absolute</Type>\n            <Path>Dialogs\\Delete Multiple Items.vi</Path>\n          </Item2Launch>\n        </MenuItem>\n      </RunTimeMenu>\n    </Page>\n    <Page>\n      <Name>\n        <eng>Waveform Inputs</eng>\n        <loc>Waveform Inputs</loc>\n      </Name>\n      <DisallowRenaming>true</DisallowRenaming>\n      <DeleteProtection>true</DeleteProtection>\n      <ExcludeFromAlphabeticalOrder>true</ExcludeFromAlphabeticalOrder>\n      <GUID>165959cb-b691-43bd-9f8b-54fe62f4b534</GUID>\n      <Glyph>\n\t\t\t  <Type>To Application Data Dir</Type>\n\t\t\t  <Path>System Explorer\\Glyphs\\ChnGroup.png</Path>\n\t\t  </Glyph>\n      <Item2Launch>\n        <Type>To Common Doc Dir</Type>\n\t\t    <Path>Custom Devices\\FPGA Addon\\Windows\\FPGA Addon Configuration.lvlibp\\Addon\\Addon System Explorer\\Extra Pages\\Waveform Inputs.vi</Path>\n      </Item2Launch>\n    </Page>\n    <Page>\n      <Name>\n        <eng>Waveform Outputs</eng>\n        <loc>Waveform Outputs</loc>\n      </Name>\n      <DisallowRenaming>true</DisallowRenaming>\n      <DeleteProtection>true</DeleteProtection>\n      <ExcludeFromAlphabeticalOrder>true</ExcludeFromAlphabeticalOrder>\n      <GUID>bc66db3e-ace6-4d58-add4-89e89e885df7</GUID>\n      <Glyph>\n        <Type>To Application Data Dir</Type>\n        <Path>System Explorer\\Glyphs\\ChnGroup.png</Path>\n      </Glyph>\n      <Item2Launch>\n        <Type>To Common Doc Dir</Type>\n        <Path>Custom Devices\\FPGA Addon\\Windows\\FPGA Addon Configuration.lvlibp\\Addon\\Addon System Explorer\\Extra Pages\\Waveform Outputs.vi</Path>\n      </Item2Launch>\n    </Page>\n    <Page>\n      <Name>\n        <eng>Scalar Input</eng>\n        <loc>Scalar Input</loc>\n      </Name>\n      <GUID>9bd0c044-925c-4d1d-a44e-de3c4043858c</GUID>\n      <Glyph>\n\t\t  \t<Type>To Application Data Dir</Type>\n\t\t  \t<Path>System Explorer\\Glyphs\\default fpga channel.png</Path>\n\t\t  </Glyph>\n      <Item2Launch>\n        <Type>To Common Doc Dir</Type>\n\t\t    <Path>Custom Devices\\FPGA Addon\\Windows\\FPGA Addon Configuration.lvlibp\\Addon\\Addon System Explorer\\Extra Pages\\Scalar Input.vi</Path>\n      </Item2Launch>\n      <RunTimeMenu>\n        <MenuItem>\n          <GUID>2cd33a82-ccc0-4cb3-affc-1385b5dc0dd8</GUID>\n          <Type>Action</Type>\n          <Name>\n            <eng>Enable Bitpacked</eng>\n            <loc>Enable Bitpacked</loc>\n          </Name>\n          <Item2Launch>\n            <Type>To Common Doc Dir</Type>\n            <Path>Custom Devices\\FPGA Addon\\Windows\\FPGA Addon Configuration.lvlibp\\Addon\\Addon System Explorer\\RTMs\\Switch Scalar Type.vi</Path>\n          </Item2Launch>\n        </MenuItem>\n        <MenuItem>\n          <GUID>7755077A-1485-13A6-5674A23FB86277FF</GUID>\n          <Type>Separator</Type>\n          <Name>\n            <eng>.</eng>\n            <loc>.</loc>\n          </Name>\n          <Item2Launch>\n            <Type>Absolute</Type>\n            <Path>.</Path>\n          </Item2Launch>\n        </MenuItem>\n        <MenuItem>\n          <GUID>77550670-1485-13A6-568B9AB41979630D</GUID>\n          <Type>Action</Type>\n          <Name>\n            <eng>Delete</eng>\n            <loc>Delete</loc>\n          </Name>\n          <Item2Launch>\n            <Type>Absolute</Type>\n            <Path>Actions\\Delete.vi</Path>\n          </Item2Launch>\n        </MenuItem>\n      </RunTimeMenu>\n    </Page>\n    <Page>\n      <Name>\n        <eng>Scalar Output</eng>\n        <loc>Scalar Output</loc>\n      </Name>\n      <GUID>625afbbf-e929-46eb-93d1-fe7033ba1e7b</GUID>\n      <Glyph>\n\t\t  \t<Type>To Application Data Dir</Type>\n\t\t  \t<Path>System Explorer\\Glyphs\\default fpga channel.png</Path>\n\t  \t</Glyph>\n      <Item2Launch>\n        <Type>To Common Doc Dir</Type>\n\t\t    <Path>Custom Devices\\FPGA Addon\\Windows\\FPGA Addon Configuration.lvlibp\\Addon\\Addon System Explorer\\Extra Pages\\Scalar Output.vi</Path>\n      </Item2Launch>\n      <RunTimeMenu>\n        <MenuItem>\n          <GUID>2cd33a82-ccc0-4cb3-affc-1385b5dc0dd8</GUID>\n          <Type>Action</Type>\n          <Name>\n            <eng>Enable Bitpacked</eng>\n            <loc>Enable Bitpacked</loc>\n          </Name>\n          <Item2Launch>\n            <Type>To Common Doc Dir</Type>\n            <Path>Custom Devices\\FPGA Addon\\Windows\\FPGA Addon Configuration.lvlibp\\Addon\\Addon System Explorer\\RTMs\\Switch Scalar Type.vi</Path>\n          </Item2Launch>\n        </MenuItem>\n        <MenuItem>\n          <GUID>7755077A-1485-13A6-5674A23FB86277FF</GUID>\n          <Type>Separator</Type>\n          <Name>\n            <eng>.</eng>\n            <loc>.</loc>\n          </Name>\n          <Item2Launch>\n            <Type>Absolute</Type>\n            <Path>.</Path>\n          </Item2Launch>\n        </MenuItem>\n        <MenuItem>\n          <GUID>77550670-1485-13A6-568B9AB41979630D</GUID>\n          <Type>Action</Type>\n          <Name>\n            <eng>Delete</eng>\n            <loc>Delete</loc>\n          </Name>\n          <Item2Launch>\n            <Type>Absolute</Type>\n            <Path>Actions\\Delete.vi</Path>\n          </Item2Launch>\n        </MenuItem>\n      </RunTimeMenu>\n    </Page>\n    <Page>\n      <Name>\n        <eng>DMA</eng>\n        <loc>DMA</loc>\n      </Name>\n      <ExcludeFromAlphabeticalOrder>true</ExcludeFromAlphabeticalOrder>\n      <GUID>fdfaa619-d09f-452b-8143-c1a261c13b7a</GUID>\n      <Glyph>\n\t\t\t  <Type>To Application Data Dir</Type>\n\t\t\t  <Path>System Explorer\\Glyphs\\Lookup Table.png</Path>\n\t\t  </Glyph>\n      <Item2Launch>\n        <Type>To Common Doc Dir</Type>\n\t\t    <Path>Custom Devices\\FPGA Addon\\Windows\\FPGA Addon Configuration.lvlibp\\Addon\\Addon System Explorer\\Extra Pages\\DMA Channel.vi</Path>\n      </Item2Launch>\n      <RunTimeMenu>\n         <MenuItem>\n            <GUID>345ad323-e622-4d27-9f97-b3d588c29827</GUID>\n            <Type>Action</Type>\n            <Name>\n              <eng>Import DMA Channels</eng>\n              <loc>Import DMA Channels</loc>\n            </Name>\n            <Item2Launch>\n              <Type>To Common Doc Dir</Type>\n              <Path>Custom Devices\\FPGA Addon\\Windows\\FPGA Addon Configuration.lvlibp\\Addon\\Addon System Explorer\\RTMs\\Import DMA Channels RTM.vi</Path>\n            </Item2Launch>\n          </MenuItem>\n          <MenuItem>\n            <GUID>7755077A-1485-13A6-5674A23FB86277FF</GUID>\n            <Type>Separator</Type>\n            <Name>\n              <eng>.</eng>\n              <loc>.</loc>\n            </Name>\n            <Item2Launch>\n              <Type>Absolute</Type>\n              <Path>.</Path>\n            </Item2Launch>\n          </MenuItem>\n      </RunTimeMenu>\n    <ButtonList>\n        <Button>\n          <ID>Import DMA Channels</ID>\n          <Glyph>\n            <Type>To Application Data Dir</Type>\n            <Path>System Explorer\\Glyphs\\NI-XNET ImportXNETFrames.png</Path>\n          </Glyph>\n          <Type>Action</Type>\n          <ReferencedGUID>345ad323-e622-4d27-9f97-b3d588c29827</ReferencedGUID>\n          <ButtonText>\n            <eng>Import DMA Channels</eng>\n            <loc>Import DMA Channels</loc>\n          </ButtonText>\n          <Caption>\n            <eng>Import DMA Channels</eng>\n            <loc>Import DMA Channels</loc>\n          </Caption>\n          <TipStrip>\n            <eng>Import DMA Channels</eng>\n            <loc>Import DMA Channels</loc>\n          </TipStrip>\n          <Documentation>\n            <eng/>\n            <loc/>\n          </Documentation>\n        </Button>\n    </ButtonList>\n    </Page>\n    <Page>\n      <Name>\n        <eng>Waveform Output</eng>\n        <loc>Waveform Output</loc>\n      </Name>\n      <DeleteProtection>true</DeleteProtection>\n      <ExcludeFromAlphabeticalOrder>true</ExcludeFromAlphabeticalOrder>\n      <GUID>0c0ecc88-7768-47db-a589-856e32a93156</GUID>\n      <Glyph>\n        <Type>To Application Data Dir</Type>\n        <Path>System Explorer\\Glyphs\\waveform.png</Path>\n      </Glyph>\n      <Item2Launch>\n        <Type>To Common Doc Dir</Type>\n        <Path>Custom Devices\\FPGA Addon\\Windows\\FPGA Addon Configuration.lvlibp\\Addon\\Addon System Explorer\\Extra Pages\\Waveform Output.vi</Path>\n      </Item2Launch>\n    </Page>\n    <Page>\n      <Name>\n        <eng>Waveform Input</eng>\n        <loc>Waveform Input</loc>\n      </Name>\n      <DeleteProtection>true</DeleteProtection>\n      <ExcludeFromAlphabeticalOrder>true</ExcludeFromAlphabeticalOrder>\n      <GUID>2afc1de4-b056-47bb-a2ad-eec5ad0d30b6</GUID>\n      <Glyph>\n        <Type>To Application Data Dir</Type>\n        <Path>System Explorer\\Glyphs\\waveform.png</Path>\n      </Glyph>\n      <Item2Launch>\n        <Type>To Common Doc Dir</Type>\n        <Path>Custom Devices\\FPGA Addon\\Windows\\FPGA Addon Configuration.lvlibp\\Addon\\Addon System Explorer\\Extra Pages\\Waveform Input.vi</Path>\n      </Item2Launch>\n    </Page>\n    <Page>\n      <Name>\n        <eng>DMA Status Channels</eng>\n        <loc>DMA Status Channels</loc>\n      </Name>\n      <DisallowRenaming>true</DisallowRenaming>\n      <DeleteProtection>true</DeleteProtection>\n      <ExcludeFromAlphabeticalOrder>true</ExcludeFromAlphabeticalOrder>\n      <GUID>4e1a084b-2b8b-4128-8417-f0007d9ffe93</GUID>\n      <Glyph>\n\t\t  \t<Type>To Application Data Dir</Type>\n\t\t  \t<Path>System Explorer\\Glyphs\\event-based.png</Path>\n\t\t  </Glyph>\n      <Item2Launch>\n        <Type>To Common Doc Dir</Type>\n\t    \t<Path>Custom Devices\\FPGA Addon\\Windows\\FPGA Addon Configuration.lvlibp\\Addon\\Addon System Explorer\\Extra Pages\\DMA Status Channels.vi</Path>\n      </Item2Launch>\n    </Page>\n    <Page>\n      <Name>\n        <eng>DMA Error</eng>\n        <loc>DMA Error</loc>\n      </Name>\n      <DisallowRenaming>true</DisallowRenaming>\n      <DeleteProtection>true</DeleteProtection>\n      <GUID>708ff167-b4eb-405e-bb0f-5c2fb305da21</GUID>\n      <Glyph>\n        <Type>To Application Data Dir</Type>\n        <Path>System Explorer\\Glyphs\\RM Information Channels.png</Path>\n      </Glyph>\n      <Item2Launch>\n        <Type>To Common Doc Dir</Type>\n        <Path>Custom Devices\\FPGA Addon\\Windows\\FPGA Addon Configuration.lvlibp\\Addon\\Addon System Explorer\\Extra Pages\\DMA Error.vi</Path>\n      </Item2Launch>\n    </Page>\n    <Page>\n      <Name>\n        <eng>DMA Elements Remaining</eng>\n        <loc>DMA Elements Remaining</loc>\n      </Name>\n      <DisallowRenaming>true</DisallowRenaming>\n      <DeleteProtection>true</DeleteProtection>\n      <GUID>785497d1-fc1e-46c9-8feb-aa61f2850cff</GUID>\n      <Glyph>\n        <Type>To Application Data Dir</Type>\n        <Path>System Explorer\\Glyphs\\RM Information Channels.png</Path>\n      </Glyph>\n      <Item2Launch>\n        <Type>To Common Doc Dir</Type>\n        <Path>Custom Devices\\FPGA Addon\\Windows\\FPGA Addon Configuration.lvlibp\\Addon\\Addon System Explorer\\Extra Pages\\DMA Elements Remaining.vi</Path>\n      </Item2Launch>\n    </Page>\n    <Page>\n      <Name>\n        <eng>Scalar Input Bitpacked</eng>\n        <loc>Scalar Input Bitpacked</loc>\n      </Name>\n      <ExcludeFromAlphabeticalOrder>true</ExcludeFromAlphabeticalOrder>\n      <GUID>8489bf21-57e3-4e68-bdd5-eadff573ec1e</GUID>\n      <Glyph>\n        <Type>To Common Doc Dir</Type>\n\t\t  <Path>Custom Devices\\FPGA Addon\\Windows\\Glyphs\\Bitpacked.png</Path>\n      </Glyph>\n      <Item2Launch>\n        <Type>To Common Doc Dir</Type>\n        <Path>Custom Devices\\FPGA Addon\\Windows\\FPGA Addon Configuration.lvlibp\\Addon\\Addon System Explorer\\Extra Pages\\Scalar Bitpacked.vi</Path>\n      </Item2Launch>\n      <RunTimeMenu>\n        <MenuItem>\n          <GUID>2cd33a82-ccc0-4cb3-affc-1385b5dc0dd8</GUID>\n          <Type>Action</Type>\n          <Name>\n            <eng>Disable Bitpacked</eng>\n            <loc>Disable Bitpacked</loc>\n          </Name>\n          <Item2Launch>\n            <Type>To Common Doc Dir</Type>\n            <Path>Custom Devices\\FPGA Addon\\Windows\\FPGA Addon Configuration.lvlibp\\Addon\\Addon System Explorer\\RTMs\\Switch Scalar Type.vi</Path>\n          </Item2Launch>\n        </MenuItem>\n        <MenuItem>\n          <GUID>7755077A-1485-13A6-5674A23FB86277FF</GUID>\n          <Type>Separator</Type>\n          <Name>\n            <eng>.</eng>\n            <loc>.</loc>\n          </Name>\n          <Item2Launch>\n            <Type>Absolute</Type>\n            <Path>.</Path>\n          </Item2Launch>\n        </MenuItem>\n        <MenuItem>\n          <GUID>77550670-1485-13A6-568B9AB41979630D</GUID>\n          <Type>Action</Type>\n          <Name>\n            <eng>Delete</eng>\n            <loc>Delete</loc>\n          </Name>\n          <Item2Launch>\n            <Type>Absolute</Type>\n            <Path>Actions\\Delete.vi</Path>\n          </Item2Launch>\n        </MenuItem>\n      </RunTimeMenu>\n    </Page>\n    <Page>\n      <Name>\n        <eng>Scalar Output Bitpacked</eng>\n        <loc>Scalar Output Bitpacked</loc>\n      </Name>\n      <ExcludeFromAlphabeticalOrder>true</ExcludeFromAlphabeticalOrder>\n      <GUID>ebfc3e29-7579-49df-b828-0da2c3787b5f</GUID>\n      <Glyph>\n        <Type>To Common Doc Dir</Type>\n\t\t  <Path>Custom Devices\\FPGA Addon\\Windows\\Glyphs\\Bitpacked.png</Path>\n      </Glyph>\n      <Item2Launch>\n        <Type>To Common Doc Dir</Type>\n        <Path>Custom Devices\\FPGA Addon\\Windows\\FPGA Addon Configuration.lvlibp\\Addon\\Addon System Explorer\\Extra Pages\\Scalar Bitpacked.vi</Path>\n      </Item2Launch>\n      <RunTimeMenu>\n        <MenuItem>\n          <GUID>2cd33a82-ccc0-4cb3-affc-1385b5dc0dd8</GUID>\n          <Type>Action</Type>\n          <Name>\n            <eng>Disable Bitpacked</eng>\n            <loc>Disable Bitpacked</loc>\n          </Name>\n          <Item2Launch>\n            <Type>To Common Doc Dir</Type>\n            <Path>Custom Devices\\FPGA Addon\\Windows\\FPGA Addon Configuration.lvlibp\\Addon\\Addon System Explorer\\RTMs\\Switch Scalar Type.vi</Path>\n          </Item2Launch>\n        </MenuItem>\n        <MenuItem>\n          <GUID>7755077A-1485-13A6-5674A23FB86277FF</GUID>\n          <Type>Separator</Type>\n          <Name>\n            <eng>.</eng>\n            <loc>.</loc>\n          </Name>\n          <Item2Launch>\n            <Type>Absolute</Type>\n            <Path>.</Path>\n          </Item2Launch>\n        </MenuItem>\n        <MenuItem>\n          <GUID>77550670-1485-13A6-568B9AB41979630D</GUID>\n          <Type>Action</Type>\n          <Name>\n            <eng>Delete</eng>\n            <loc>Delete</loc>\n          </Name>\n          <Item2Launch>\n            <Type>Absolute</Type>\n            <Path>Actions\\Delete.vi</Path>\n          </Item2Launch>\n        </MenuItem>\n      </RunTimeMenu>\n    </Page>\n    <Page>\n      <Name>\n        <eng>Bitpacked Input</eng>\n        <loc>Bitpacked Input</loc>\n      </Name>\n      <DeleteProtection>true</DeleteProtection>\n      <ExcludeFromAlphabeticalOrder>true</ExcludeFromAlphabeticalOrder>\n      <GUID>4b03cffd-e469-431a-ba96-aca85ece66af</GUID>\n      <Glyph>\n        <Type>To Application Data Dir</Type>\n        <Path>System Explorer\\Glyphs\\default fpga channel.png</Path>\n      </Glyph>\n      <Item2Launch>\n        <Type>To Common Doc Dir</Type>\n        <Path>Custom Devices\\FPGA Addon\\Windows\\FPGA Addon Configuration.lvlibp\\Addon\\Addon System Explorer\\Extra Pages\\Scalar Input.vi</Path>\n      </Item2Launch>\n    </Page>\n    <Page>\n      <Name>\n        <eng>Bitpacked Output</eng>\n        <loc>Bitpacked Output</loc>\n      </Name>\n      <DeleteProtection>true</DeleteProtection>\n      <ExcludeFromAlphabeticalOrder>true</ExcludeFromAlphabeticalOrder>\n      <GUID>6db3f02b-654f-4ed6-bd84-80bb5242a557</GUID>\n      <Glyph>\n        <Type>To Application Data Dir</Type>\n        <Path>System Explorer\\Glyphs\\default fpga channel.png</Path>\n      </Glyph>\n      <Item2Launch>\n        <Type>To Common Doc Dir</Type>\n        <Path>Custom Devices\\FPGA Addon\\Windows\\FPGA Addon Configuration.lvlibp\\Addon\\Addon System Explorer\\Extra Pages\\Scalar Output.vi</Path>\n      </Item2Launch>\n    </Page>\n      <Page>\n      <Name>\n        <eng>Static Scalar Input</eng>\n        <loc>Static Scalar Input</loc>\n      </Name>\n      <GUID>7579cb69-d559-4b2b-a1fc-0d112e8661b6</GUID>\n      <Glyph>\n        <Type>To Application Data Dir</Type>\n        <Path>System Explorer\\Glyphs\\default fpga channel.png</Path>\n      </Glyph>\n      <Item2Launch>\n        <Type>To Common Doc Dir</Type>\n        <Path>Custom Devices\\FPGA Addon\\Windows\\FPGA Addon Configuration.lvlibp\\Addon\\Addon System Explorer\\Extra Pages\\Scalar Input.vi</Path>\n      </Item2Launch>\n      <RunTimeMenu>\n        <MenuItem>\n          <GUID>77550670-1485-13A6-568B9AB41979630D</GUID>\n          <Type>Action</Type>\n          <Name>\n            <eng>Delete</eng>\n            <loc>Delete</loc>\n          </Name>\n          <Item2Launch>\n            <Type>Absolute</Type>\n            <Path>Actions\\Delete.vi</Path>\n          </Item2Launch>\n        </MenuItem>\n      </RunTimeMenu>\n    </Page>\n    <Page>\n      <Name>\n        <eng>Static Scalar Output</eng>\n        <loc>Static Scalar Output</loc>\n      </Name>\n      <GUID>ddc5186b-4b14-4629-b48a-cef4575f789c</GUID>\n      <Glyph>\n        <Type>To Application Data Dir</Type>\n        <Path>System Explorer\\Glyphs\\default fpga channel.png</Path>\n      </Glyph>\n      <Item2Launch>\n        <Type>To Common Doc Dir</Type>\n        <Path>Custom Devices\\FPGA Addon\\Windows\\FPGA Addon Configuration.lvlibp\\Addon\\Addon System Explorer\\Extra Pages\\Scalar Output.vi</Path>\n      </Item2Launch>\n      <RunTimeMenu>\n        <MenuItem>\n          <GUID>77550670-1485-13A6-568B9AB41979630D</GUID>\n          <Type>Action</Type>\n          <Name>\n            <eng>Delete</eng>\n            <loc>Delete</loc>\n          </Name>\n          <Item2Launch>\n            <Type>Absolute</Type>\n            <Path>Actions\\Delete.vi</Path>\n          </Item2Launch>\n        </MenuItem>\n      </RunTimeMenu>\n    </Page>\n      <Page>\n      <Name>\n        <eng>Speciality IO</eng>\n        <loc>Speciality IO</loc>\n      </Name>\n      <ExcludeFromAlphabeticalOrder>true</ExcludeFromAlphabeticalOrder>\n      <GUID>25832021-24b6-475a-aa84-f4ed7870ed99</GUID>\n      <Glyph>\n        <Type>To Common Doc Dir</Type>\n\t\t  <Path>Custom Devices\\FPGA Addon\\Windows\\Glyphs\\IP Core.png</Path>\n      </Glyph>\n      <Item2Launch>\n        <Type>To Common Doc Dir</Type>\n        <Path>Custom Devices\\FPGA Addon\\Windows\\FPGA Addon Configuration.lvlibp\\Addon\\Addon System Explorer\\Extra Pages\\Speciality IO.vi</Path>\n      </Item2Launch>\n    </Page>\n  </Pages>\n  <CustomXML>\n    <Dummy/>\n  </CustomXML>\n</CustomDevice>"] ("Array") -> [w33] mode=indexing
        tunnel: [w28] -> w14
        tunnel: w11 -> [w26]
        tunnel: w10 -> [w25] mode=indexing
        tunnel: [w25] -> w8
        tunnel: w5 -> [w23]
        stop <- w31 stop-if-true
        # "UUT"
        n6 = Build Path(base path=w26, name or relative path=w25) -> (appended path=w27:path)
        n7 = call "Update Custom Device XML.vi"("Build Spec Type"=w37, "error in (no error)"=w29, "CD XML/Project Path"=w36, "Packed Library Path"=w27) -> ("error out"=w34:errorcluster, "Project XML Editor out"=w24:refnum<class "Project XML Editor.lvclass">)  [unwired: 6 in]
        n8 = call "Destroy XML Editor.vi"("error in (no error)"=w34, "Project XML Editor in"=w24) -> ("error out"=w35:errorcluster)  [unwired: 9 in]
        n9 = Read from Text File(file (use dialog)=w23, error in=w35) -> (text=w32:string, error out=w30:errorcluster)  [unwired: 2 in, 2 out]
        n10 = Not Equal?(x=w33, y=w32) -> (x != y?=w28:bool)
        n11 = Or(x=w28, y=w30) -> (x .or. y?=w31:bool)
      }
      n12 = Concatenate Strings("Error during the CD XML update process for the following library:" ("message (\"\")"), w8) -> (w12:string)
      n13 = call-dynamic "failIf.vi"("error in (no error)"=w7, "message (\"\")"=w12, "fail"=w14, "TestCase in"=w16) -> ("error out"=w6:errorcluster, "TestCase out"=w15:refnum<class "LVLIBP CD XML Updater Unit Tests.lvclass">)  [unwired: 6 in]
    }
    frame Disabled {
      # "skip test result while test is under development"
      n14 = call <vilib>:"skip.vi"("error in (no error)"=w38, "TestCase in"=w41) -> ("error out"=w40:errorcluster, "TestCase out"=w39:refnum<class "LVLIBP CD XML Updater Unit Tests.lvclass">)  [unwired: 8 in]
    }
  }
  "error out" <- w3
  "TestCase out" <- w1
